vi "CRYGraph Property Window Polar.vi"(9 "TabName":string, 10 "Graph VI Ref":refnum<vi>) -> ()   [LabVIEW 2013]
uses:
  Control/CRYPolar Property.ctl
  <vilib>/Utility/miscctls.llb/LVRowAndColumnTypeDef.ctl
  CRYCurveLibrary/Global/CRYCurve Library Global.vi
panel:
  in  "Dis/RanFreqUpdate":bool
  in  "XYCursorChange":string caption="Title Name"
  in  "EndbyOK":bool
  in  "FreqUpdate":bool
  out "Scale Style":u8=5
  out "Interpolation":string
  in  "Plot PropertyCtrl Ref":refnum<vi>
  in  "Plot Property":string
  out "PointStyle":string
  out "LineWidth":string
  out "LineStyle":string
  out "CurValuesRef":refnum<vi>[](array[refnum])
  out "CruColorsRef":refnum<vi>[](array[refnum])
  in  "SetFormat":bool
  in  "No Data":bool
  in  "CurColValPlot":bool
  out "CurColors":u32[](array[numeric])
  out "CurValues":dbl[](array[numeric])
  in  "Draw":bool
  in  "Polar Property":T1={"polar attributes"={"maximum"=2.0, "minimum"=0.0, "clip to min"=FALSE, "log"=FALSE, "grid color"=3381657, "plot color"=16711680, "fmt and prec"={"format"=enum."Decimal", "precision"=2}, "visible section"=4}, "Auto/Manual"=0, "Zero Adjust (deg)"=0, "Angle Increment (deg)"=0, "Mirror"=FALSE, "Auto Increment"=FALSE, "Total Rotatin (deg)"=0, "Discrete/Rannge"=0, "Show Name"=FALSE, "CurValues"=[], "CurIndex"=0, "CurColors"=[], "CurColors_Range"=[], "CurValues_Range"=[], "Pen"={"Width"=1, "Style"=enum."Solid"}, "BackgroundColor"=0} {"polar attributes"."minimum" format="%0.2f"; "polar attributes"."maximum" format="%0.2f"}
  in  "Polar Tab":enum32{"Title", "Plot", "XY Graph"}(tab)
  in  "Background Color":u32(colorbox) caption="背景颜色"
  in  "Title Name":string caption="标题名字"
  out "CurValue0_1":bool
  in  "CurValue4":dbl format="%#.5p"
  in  "CurColor4":u32(colorbox)
  in  "CurValue3":dbl format="%#.5p"
  in  "CurColor3":u32(colorbox)
  in  "CurValue2":dbl format="%#.5p"
  in  "CurColor2":u32(colorbox)
  in  "CurValue1":dbl caption="末尾频率" format="%#.5p"
  in  "CurColor1":u32(colorbox)
  in  "Delete":bool
  in  "Add":bool
  in  "Show Name":bool caption="显示名字"
  out "Cursors":bool caption="游标"
  in  "Discrete/Range":u16(slide)
  in  "CurIndex":u16
  in  "CurValue0":dbl caption="开始频率" format="%#.5p"
  in  "CurColor0":u32(colorbox)
  out "Plot Options":bool caption="绘图选项"
  out "Scaling":bool caption="缩放"
  in  "Auto Increment":bool caption="自动增量"
  in  "Log":bool caption="对数"
  in  "Mirror":bool caption="镜子反射"
  in  "Auto/Manual":u16(slide)
  in  "Minimum":dbl caption="最小值"
  in  "Clip to min":bool caption="剪辑最低"
  in  "Angle Increment (deg)":i32 caption="角度增量(度)"
  in  "Zero Adjust (deg)":i32 caption="调零(度)"
  in  "Maximum":dbl caption="最大值"
  in  "PrecisionPolar":u8 caption="精度"
  in  "Grid Color":u32(colorbox) caption="网格颜色"
  in  "Line Width":u16(ring) caption="绘图线宽度" items=["1", "2", "3", "4", "5", "6"]
  in  "Visible Section":u16(ring)=4 caption="可见部分"
  in  "Total Rotatin (deg)":i32 caption="aa"
  in  "Line Style":u16(ring) caption="线条样式" items=["实线", "虚线", "点线", "点划线", "双点划线"]
  in  "PolarXY Tab":enum32{"Format and Precision", "Plot", "Scale"}(tab) caption="Property Tab"
  in  "FormatAxis":u16(ring) items=["Hz", "dB re 1 ", "dB re 1"]
  in  "NotationXY":i32(listbox)
  in  "PrecisionType":u16(ring) items=["精度位数", "有效数字"]
  in  "PrecisionDigits":u16
  in  "Hide trailing zeros":bool caption="隐藏尾随零"
  in  "Exponent in multiples of 3":bool caption="指数"
  in  "Use minimum field width":bool caption="使用最小场宽度"
  in  "Field Width":u16
  in  "PadType":u16(ring) items=["在左加空格", "在右加空格", "在左加零"]
  in  "Ignore timestamp information":bool caption="忽略时间戳信息"
  in  "TimeFormat":u16(ring) items=["Custom time format", "System time format", "Time unused"]
  in  "Digits":u16 caption="数字"
  in  "DateFormat":u16(ring) items=["Custom date format", "System date format", "Date unused"]
  in  "YMD":u16(slide)
  in  "YearShow":u16(slide)
  in  "AMFM":u16(slide)=1
  in  "HMS":u16(slide)=1
  in  "Point/Fill":u32(colorbox) caption="点/填充"
  in  "Fill to":i16(ring) caption="填写" items=["无"=-1, "零"=-2, "-无穷"=-3, "+无穷"=-4]
  in  "Items":u16(ring) items=["Crown Amp-R corr-out", "Crown Amp-R eq-out"]
  out "Colors":bool caption="颜色"
  in  "Line":u32(colorbox) caption="线"
  in  "LineStyle4":bool
  in  "LineStyle3":bool
  in  "LineStyle2":bool
  in  "LineStyle0":bool
  in  "LineStyle1":bool
  in  "LineWidth5":bool
  in  "LineWidth1":bool
  in  "LineWidth4":bool
  in  "LineWidth3":bool
  in  "LineWidth2":bool
  in  "LineWidth0":bool
  in  "PointStyle16":bool
  in  "PointStyle15":bool
  in  "PointStyle14":bool
  in  "PointStyle13":bool
  in  "PointStyle12":bool
  in  "PointStyle11":bool
  in  "PointStyle10":bool
  in  "PointStyle9":bool
  in  "PointStyle8":bool
  in  "PointStyle7":bool
  in  "PointStyle6":bool
  in  "PointStyle5":bool
  in  "PointStyle4":bool
  in  "PointStyle3":bool
  in  "PointStyle2":bool
  in  "PointStyle1":bool
  in  "PointStyle0":bool
  in  "Interpolation4":bool
  in  "Interpolation5":bool
  in  "Interpolation3":bool
  in  "Interpolation2":bool
  in  "Interpolation1":bool
  in  "Interpolation0":bool
  in  "Show Plot":bool caption="显示绘图"
  in  "GridStyle":u16(ring)=4
  out "Grid Colors":bool caption="网格颜色"
  in  "Minor grid":u32(colorbox) caption="辅网格"
  in  "Major grid":u32(colorbox) caption="主网格"
  in  "Marker text":u32(colorbox) caption="标记文本"
  in  "Minor tick":u32(colorbox) caption="辅刻度"
  in  "LogXY":bool caption="对数"
  in  "Show scale":bool caption="显示缩放"
  in  "Show scale label":bool caption="显示缩放标签"
  in  "MaximumXY":dbl caption="最大值"
  in  "MinimumXY":dbl caption="最小值"
  in  "Autoscale":bool caption="自动缩放"
  in  "Axis Name":string caption="名字"
  in  "Axis":u16(ring) items=["Hz", "dB re 1 ", "dB re 1"]
  in  "Major tick":u32(colorbox) caption="主刻度"
  out "Scale Style and Colors":bool caption="缩放样式和颜色"
  in  "OK":bool
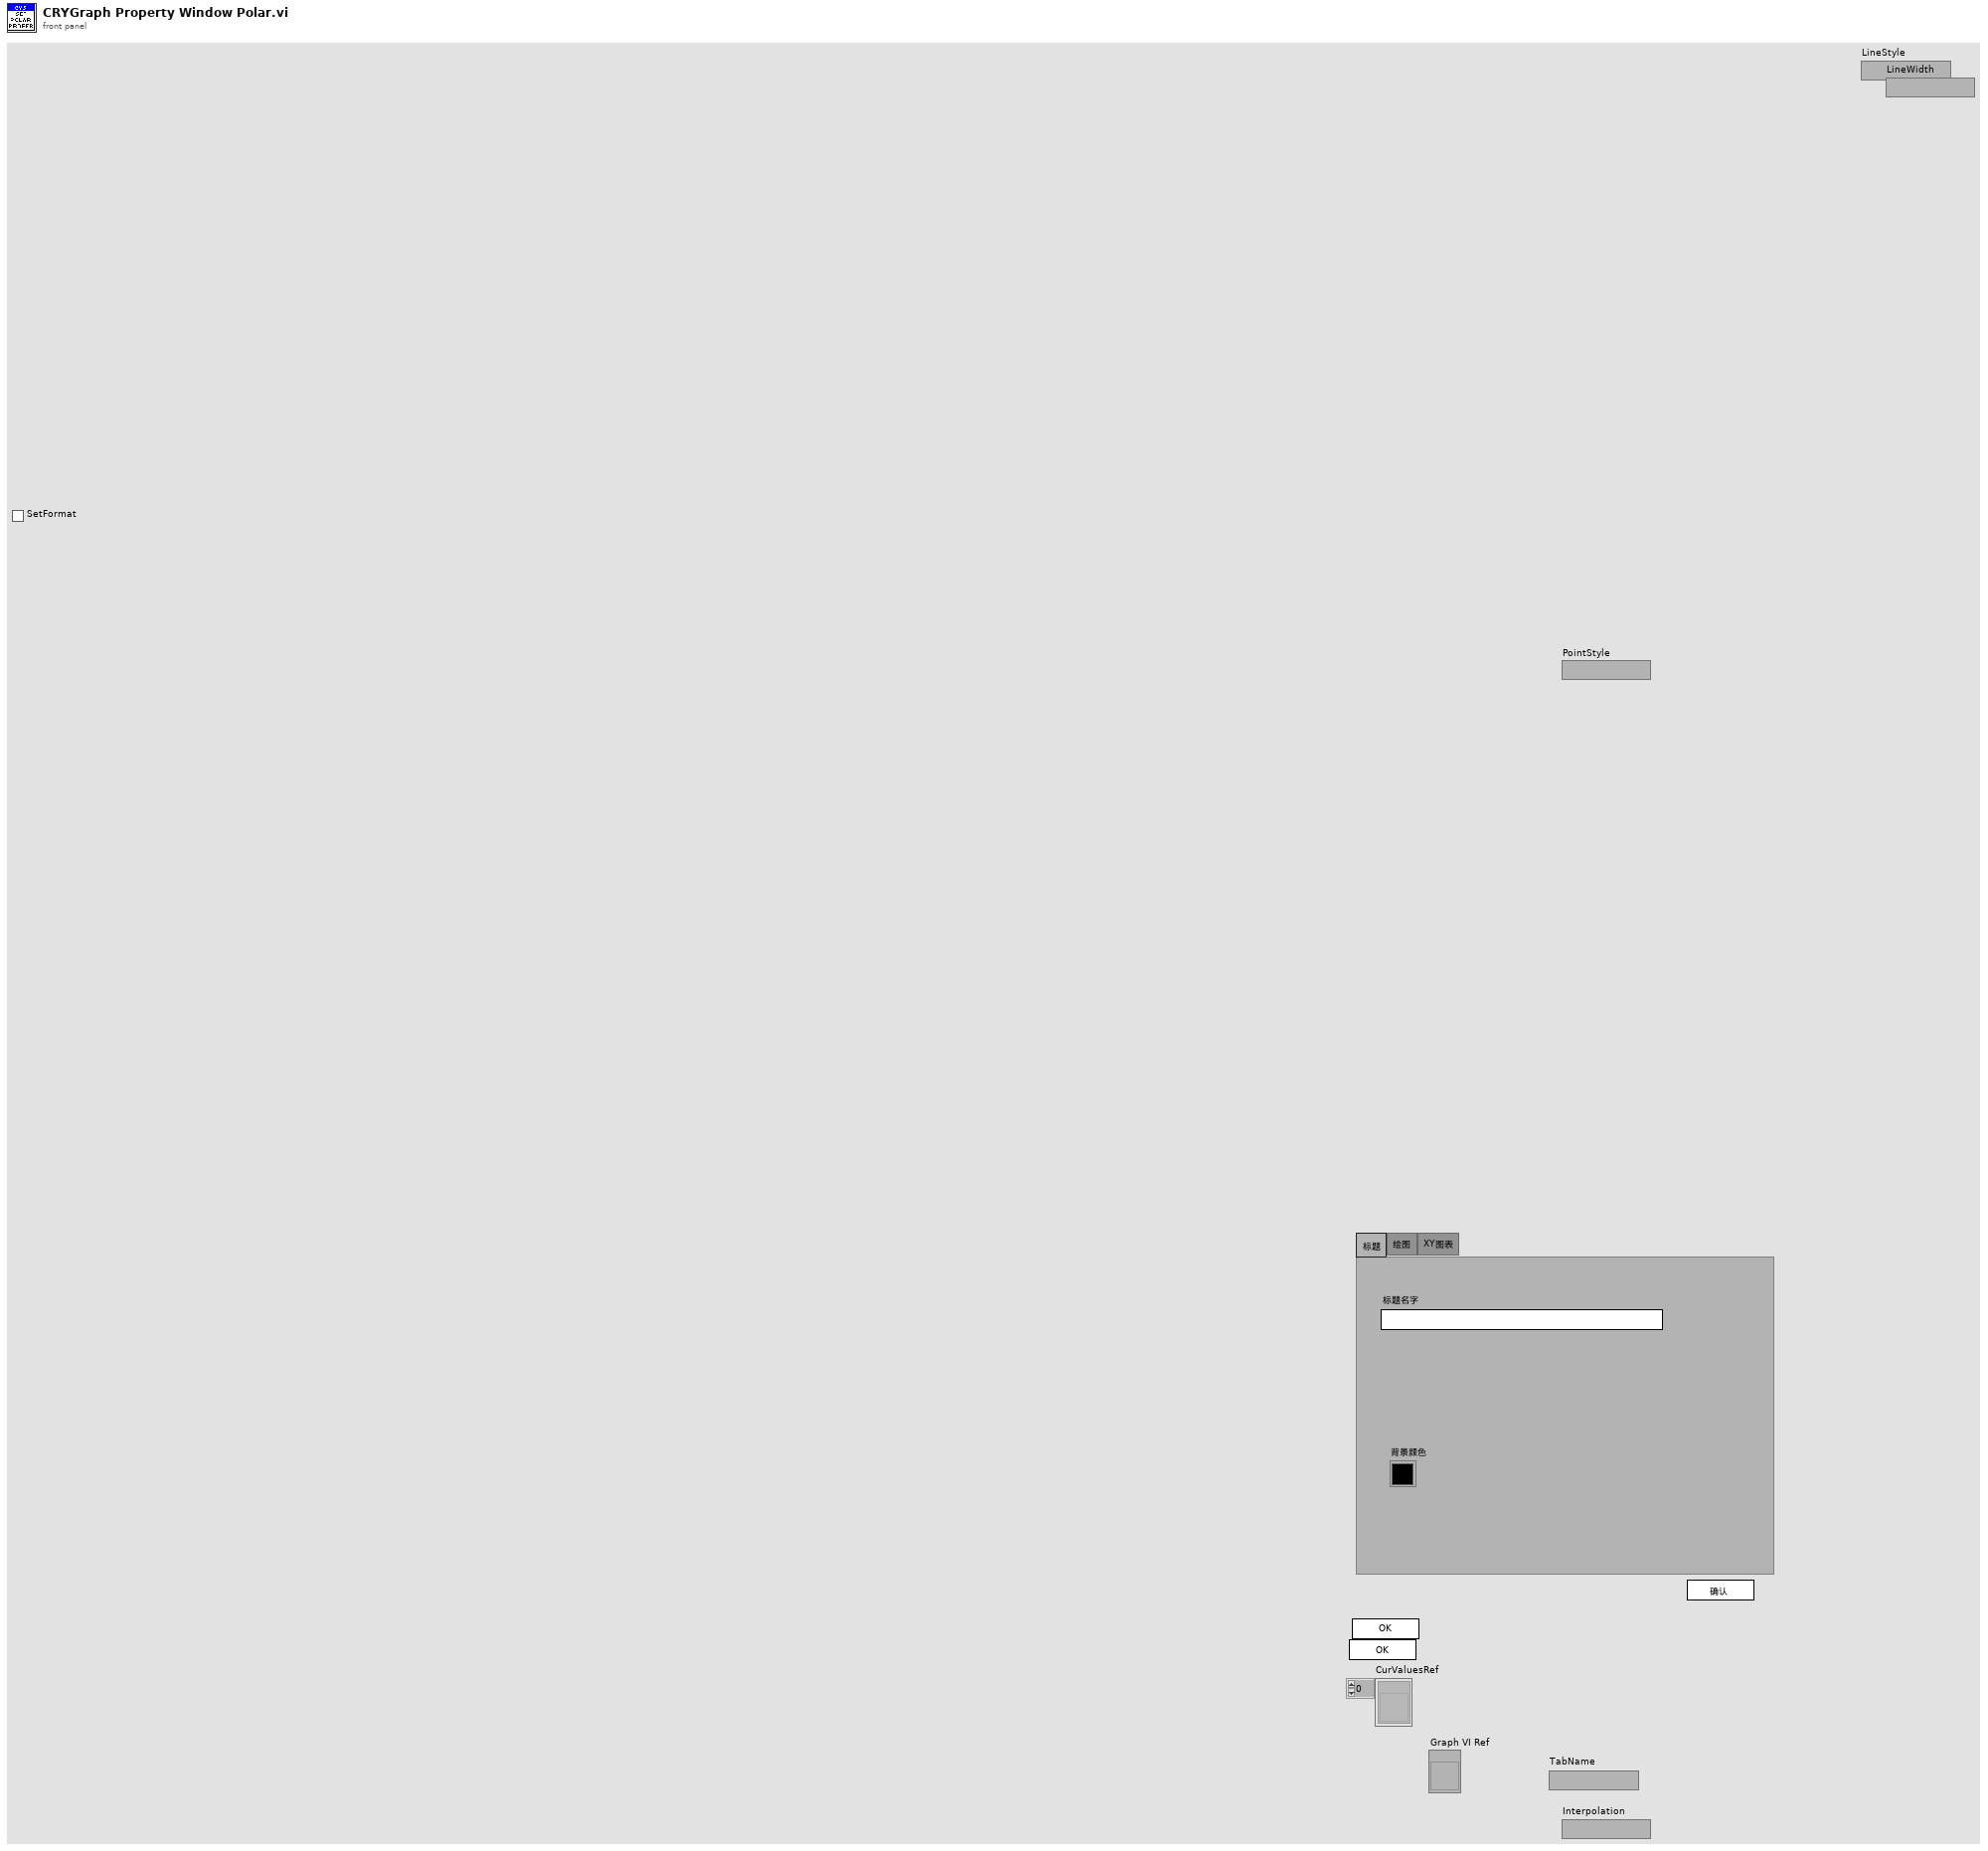
[diagram p1: front panel]
types:
  T1 = typedef "CRYPolar Property.ctl" = cluster{"polar attributes":cluster{"maximum":dbl, "minimum":dbl, "clip to min":bool, "log":bool, "grid color":u32, "plot color":u32, "fmt and prec":cluster{"format":enum8{"Decimal", "Scientific", "Engineering", "Binary", "Octal", "Hex"}, "precision":u8}, "visible section":u16}, "Auto/Manual":u16, "Zero Adjust (deg)":i32, "Angle Increment (deg)":i32, "Mirror":bool, "Auto Increment":bool, "Total Rotatin (deg)":i32, "Discrete/Rannge":u16, "Show Name":bool, "CurValues":dbl[], "CurIndex":u16, "CurColors":u32[], "CurColors_Range":u32[], "CurValues_Range":dbl[], "Pen":cluster{"Width":u16, "Style":enum32{"Solid", "Dash", "Dot", "DashDot", "DashDotDot"}}, "BackgroundColor":u32}
  T2 = enum32{"Page Enabled", "Page Disabled", "Page Disabled & Grayed"}
  T3 = enum8{"Enabled", "Disabled", "Disabled and Grayed Out"}
  T4 = typedef "LVCursorListTypeDef.ctl" = cluster{"Name":string, "Color":u32, "Style":u8, "Point Style":u8, "Name Visible":bool, "Allow Drag":bool, "Cursor Mode":u32, "Plot":i32, "Index":i32, "Position":cluster{"X":dbl, "Y":dbl}, "X Scale":u32, "Y Scale":u32, "Watch Plots":i32[], "Watch All Plots":bool, "Plot Area":i32, "Label Offset":cluster{"X":dbl, "Y":dbl}}[]
  T5 = cluster{"Width":u16, "Style":enum32{"Solid", "Dash", "Dot", "DashDot", "DashDotDot"}}
  T6 = cluster{"maximum":dbl, "minimum":dbl, "clip to min":bool, "log":bool, "grid color":u32, "plot color":u32, "fmt and prec":cluster{"format":enum8{"Decimal", "Scientific", "Engineering", "Binary", "Octal", "Hex"}, "precision":u8}, "visible section":u16}
  T7 = enum32{"Solid", "Dash", "Dot", "DashDot", "DashDotDot"}
  T8 = cluster{"format":enum8{"Decimal", "Scientific", "Engineering", "Binary", "Octal", "Hex"}, "precision":u8}
  T9 = enum16{"OK", "Yes", "YesNo", "YesNoCancel", "ReplaceAppend"}
  T10 = enum8{"Decimal", "Scientific", "Engineering", "Binary", "Octal", "Hex"}
  T11 = typedef "LVRowAndColumnTypeDef.ctl" = cluster{"Row":i32, "Column":i32}
  T12 = typedef "CRYData Cluster.ctl" = cluster{"Name":string, "Curve":cluster{"x":dbl, "y":dbl, "z":dbl}[], "X data":u16, "Y data":u16, "Z data":u16, "X axis":u16, "Y axis":u16, "Z axis":u16, "X unit":string, "Y unit":string, "Z unit":string, "X dB ref":dbl, "Y dB ref":dbl, "Z dB ref":dbl, "single val":bool, "protected":bool, "display X":bool, "display Y":bool, "display Z":bool, "Test Info":string, "Step No.":i32, "Plot Settings":cluster{"Color":u32, "Interpolation":u8, "Point Style":u8, "Line Style":u8, "Point Color":u32, "Line Width":u8, "Bar Plot Style":u8, "Fill To":i16}, "AutoProtect":bool}
  T13 = cluster{"Notation":i32, "PrecisionType":u16, "PrecisionDigits":u16, "Hide trailing zeros":bool, "Exponent in multiples of 3":bool, "Field Width":u16, "PadType":u16, "Use minimum field width":bool, "TimeFormat":u16, "AMFM":u16, "HMS":u16, "Digits":u16, "DateFormat":u16, "YMD":u16, "YearShow":u16}
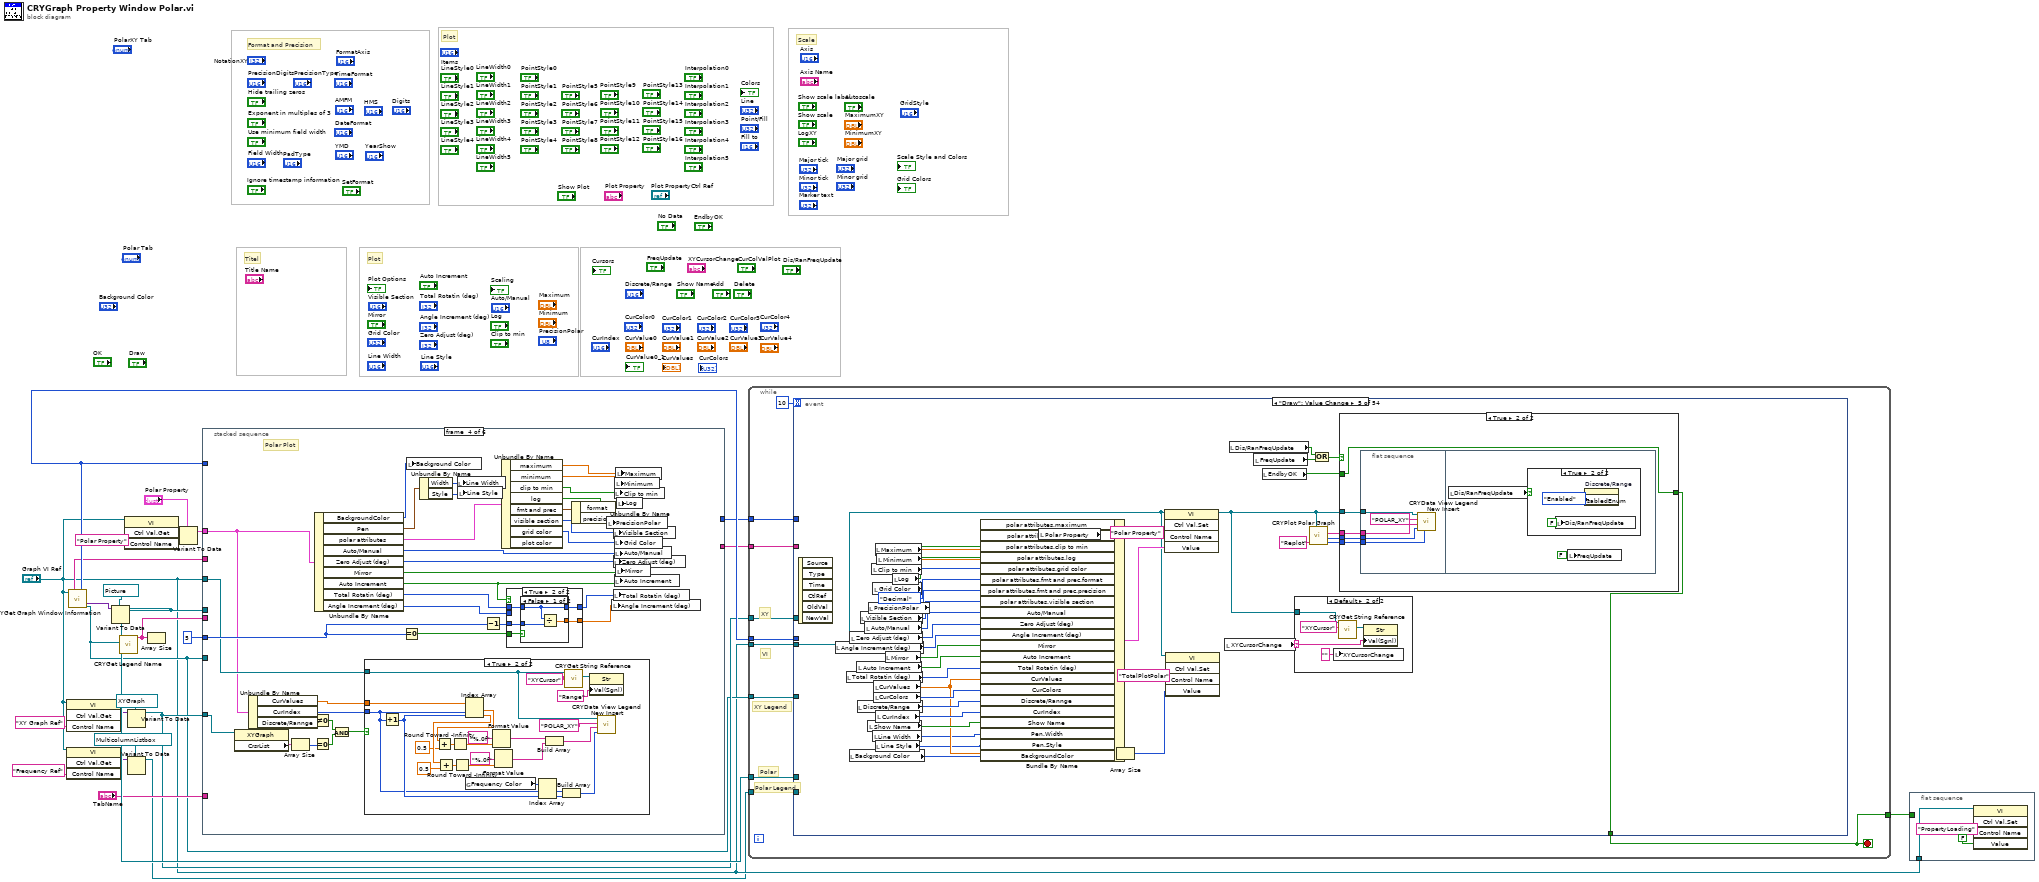
[diagram p0: block diagram]
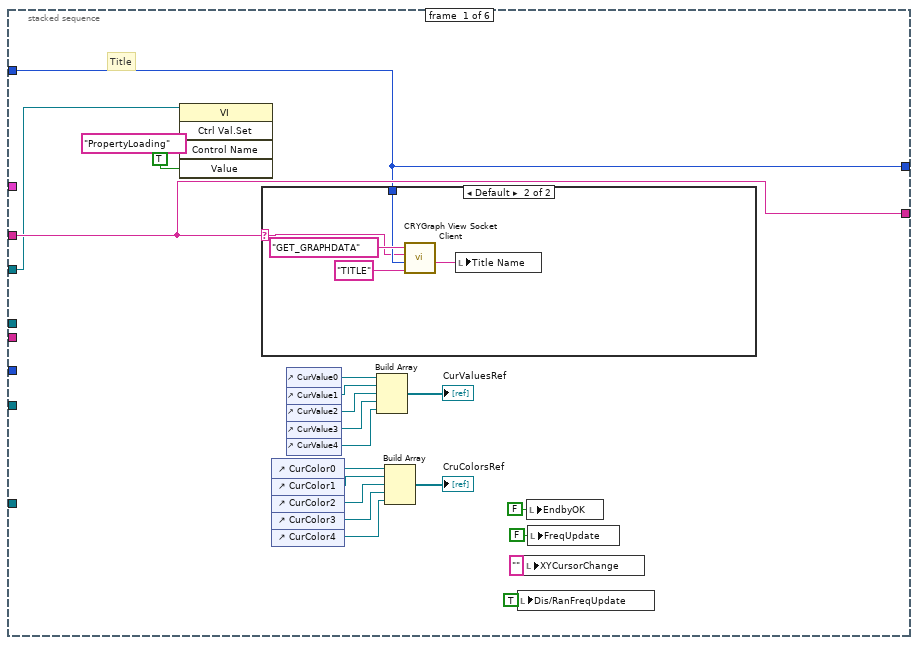
[diagram p2: hidden frame]
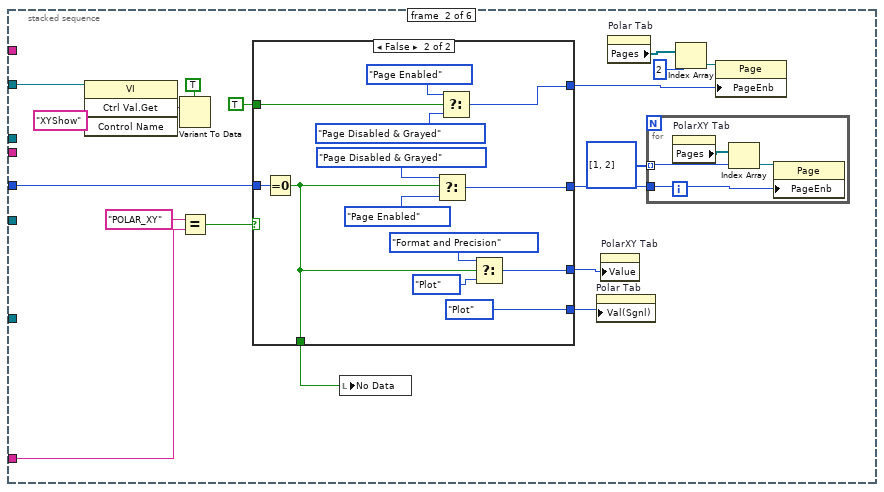
[diagram p4: hidden frame]
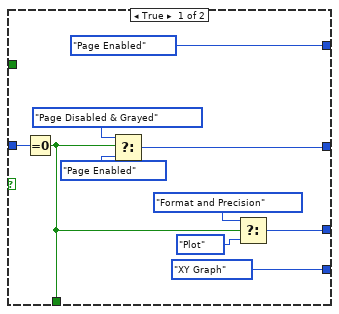
[diagram p5: hidden frame]
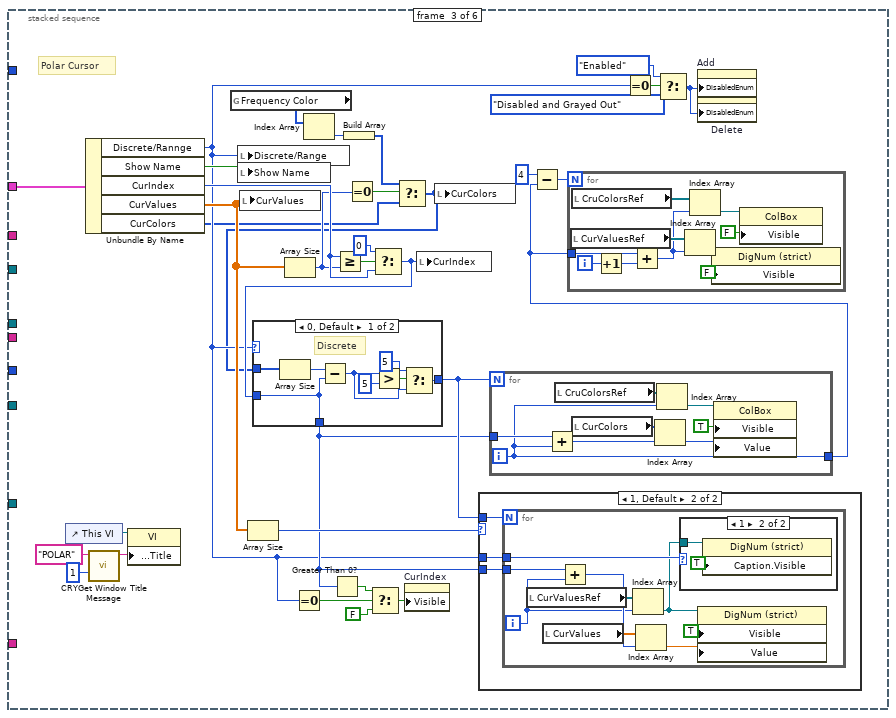
[diagram p6: hidden frame]
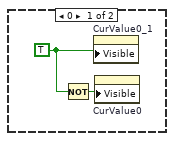
[diagram p7: hidden frame]
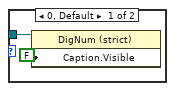
[diagram p8: hidden frame]
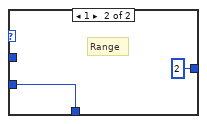
[diagram p9: hidden frame]
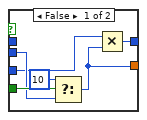
[diagram p11: hidden frame]
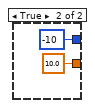
[diagram p12: hidden frame]
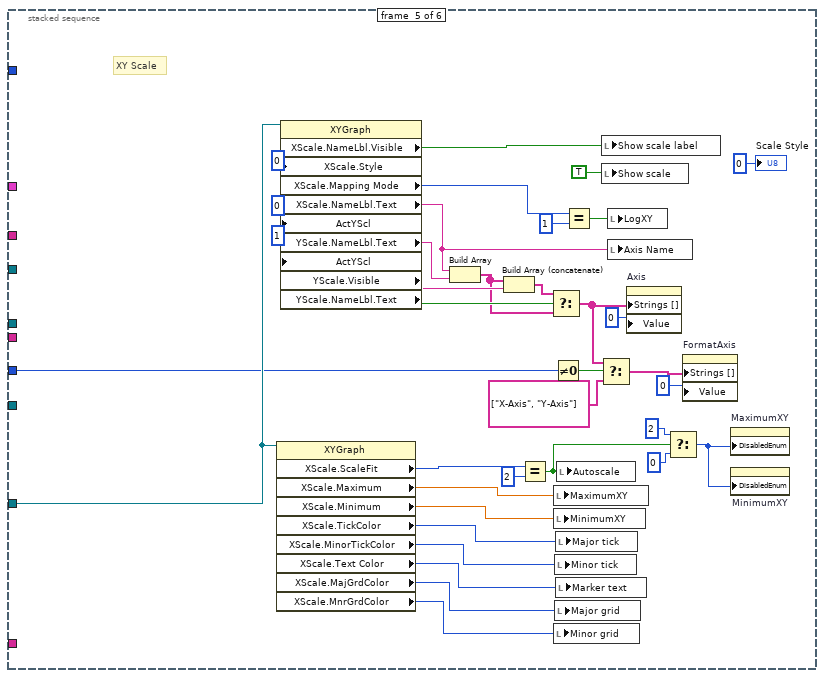
[diagram p13: hidden frame]
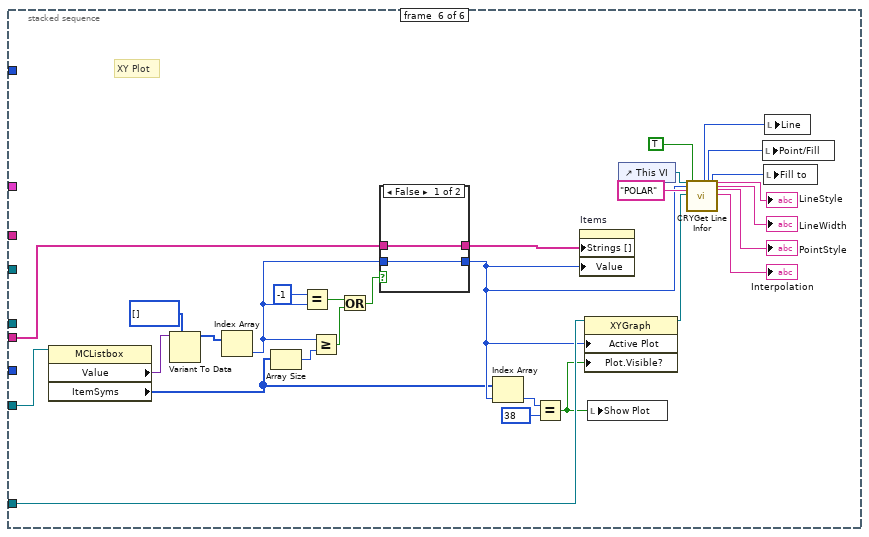
[diagram p14: hidden frame]
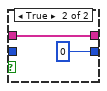
[diagram p15: hidden frame]
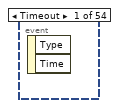
[diagram p16: hidden frame]
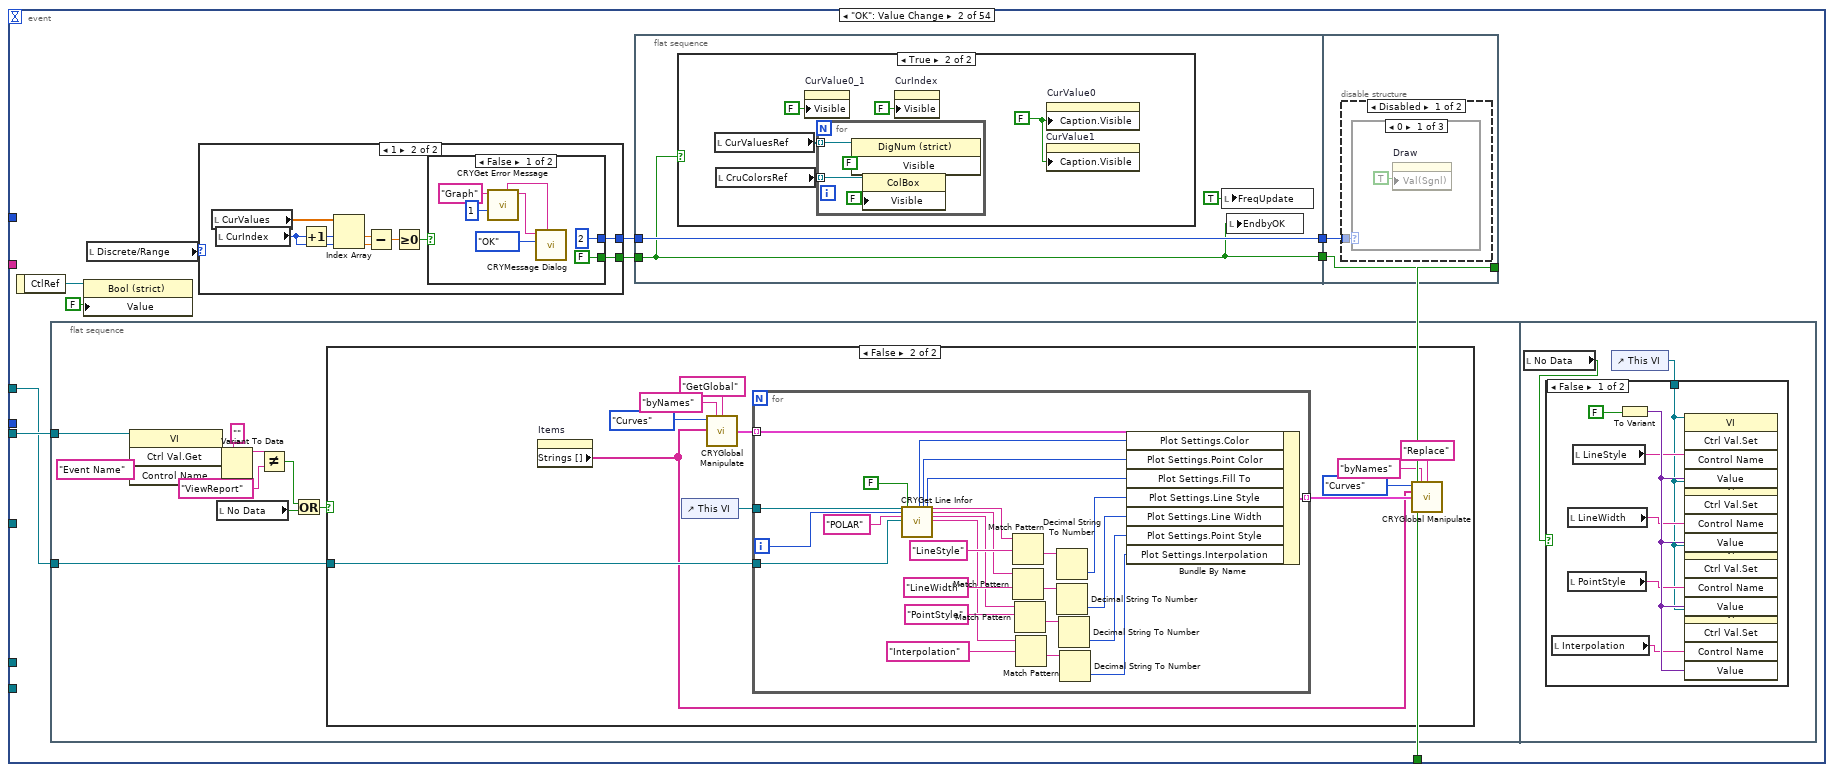
[diagram p17: hidden frame]
diagram:
  # "Format and Precision"
  # "Scale"
  # "Plot"
  # "Plot"
  # "Titel"
  n1 = invoke class="VI" method="Ctrl Val.Get"(reference="Graph VI Ref", "Control Name"="XY Graph Ref") -> ("Get Control Value Variant"=w4:variant)  [unwired: 2 in, 3 out]
  n2 = invoke class="VI" method="Ctrl Val.Get"(reference="Graph VI Ref", "Control Name"="Frequency Ref") -> ("Get Control Value Variant"=w3:variant)  [unwired: 2 in, 3 out]
  n3 = call "CRYGet Graph Window Information.vi"("pGraph VI In"="Graph VI Ref") -> ("Queue Name Out"=w23:string, "Graph Number Out"=w24:i32, "Graph Control Ref Out"=w10:variant, "Legend Ref Out"=w16:refnum<vi>)  [unwired: 2 in, 9 out]
  n4 = Variant To Data(type=refnum<vi> refnum ("Graph Ref"), Variant=w10) -> (data=w25:refnum<vi>)  [unwired: 1 in, 1 out]
  n5 = call "CRYGet Legend Name.vi"("MCListbox Refnum"=w16) -> ("Names Out"=w17:string[])  [unwired: 1 in, 9 out]
  n6 = invoke class="VI" method="Ctrl Val.Get"(reference="Graph VI Ref", "Control Name"="Polar Property") -> ("Get Control Value Variant"=w9:variant)  [unwired: 2 in, 3 out]
  n7 = Variant To Data(type=refnum<vi> refnum ("XY Graph"), Variant=w4) -> (data=w19:refnum<vi>)  [unwired: 1 in, 1 out]
  n8 = Variant To Data(type=refnum<vi> refnum ("XY Graph"), Variant=w3) -> (data=w13:refnum<vi>)  [unwired: 1 in, 1 out]
  n9 = Array Size(array=w17) -> ()  [unwired: 1 out]
  n10 = Variant To Data(type="Polar Property", Variant=w9) -> (data=w21:T1)  [unwired: 1 in, 1 out]
  n11 = stacked-sequence {
    tunnel: w25 -> [_ _ _ _ _ _]
    tunnel: w24 -> [w26 _ _ _ _ _]
    tunnel: w23 -> [w46 _ _ _ _ _]
    tunnel: [w46 _ _ _ _ _] -> w22
    tunnel: w21 -> [_ _ w129 w180 _ _]
    tunnel: "TabName" -> [_ w53 _ _ _ _]
    tunnel: "Graph VI Ref" -> [w31 w55 _ w188 _ _]
    tunnel: w19 -> [_ _ _ w187 w272 w300]
    tunnel: 5 -> [_ w54 _ w191 w253 _]
    tunnel: w17 -> [_ _ _ _ _ w302]
    tunnel: w16 -> [_ _ _ _ _ w301]
    tunnel: [w26 _ _ _ _ _] -> w12
    frame #0 {
      # "Title"
      n12 = invoke class="VI" method="Ctrl Val.Set"(reference=w31, "Control Name"="PropertyLoading", "Value"=TRUE ("FreqUpdate")) -> ()  [unwired: 2 in, 5 out]
      n13 = case shown="Default" w46 {
        selector: w46 -> [_ w48]
        tunnel: w26 -> [_ w49]
        frame "test DataView" {
        }
        frame Default {
          n14 = call "CRYGraph View Socket Client.vi"("sOption"="TITLE", "nData"=w49, "sData"=w48, "sAction"="GET_GRAPHDATA") -> ("sData Out"=w47:string)  [unwired: 4 in, 3 out]
          n15 = local write "Title Name"(w47) -> ()
        }
      }
      n16 = control-ref of="CurColor0"() -> (w45:refnum<vi>)
      n17 = control-ref of="CurColor1"() -> (w44:refnum<vi>)
      n18 = control-ref of="CurColor2"() -> (w43:refnum<vi>)
      n19 = control-ref of="CurColor3"() -> (w42:refnum<vi>)
      n20 = control-ref of="CurColor4"() -> (w41:refnum<vi>)
      n21 = control-ref of="CurValue0"() -> (w40:refnum<vi>)
      n22 = control-ref of="CurValue1"() -> (w39:refnum<vi>)
      n23 = control-ref of="CurValue2"() -> (w38:refnum<vi>)
      n24 = control-ref of="CurValue3"() -> (w37:refnum<vi>)
      n25 = control-ref of="CurValue4"() -> (w36:refnum<vi>)
      n26 = Build Array(w40, w39, w38, w37, w36) -> (→"CurValuesRef":refnum<vi>[])
      n27 = Build Array(w45, w44, w43, w42, w41) -> (→"CruColorsRef":refnum<vi>[])
      n28 = local write "Dis/RanFreqUpdate"(TRUE ("Dis/RanFreqUpdate")) -> ()
      n29 = local write "XYCursorChange"("" ("XYCursorChange")) -> ()
      n30 = local write "EndbyOK"(FALSE ("EndbyOK")) -> ()
      n31 = local write "FreqUpdate"(FALSE ("FreqUpdate")) -> ()
    }
    frame #1 {
      n32 = invoke class="VI" method="Ctrl Val.Get"(reference=w55, "Control Name"="XYShow") -> ("Get Control Value Variant"=w60:variant)  [unwired: 2 in, 3 out]
      n33 = Variant To Data(type=TRUE, Variant=w60) -> ()  [unwired: 1 in, 2 out]
      n34 = Equal?(x="POLAR_XY" ("y"), y=w53) -> (x = y?=w67:bool)
      n35 = case shown="False" w67 {
        tunnel: TRUE -> [_ w89]
        tunnel: [enum32{"Title", "Plot", "XY Graph"}."XY Graph" ("Value (Signaling)") enum32{"Title", "Plot", "XY Graph"}."Plot" ("Value (Signaling)")] -> w66
        tunnel: w54 -> [w82 w95]
        tunnel: [w79 w92] -> w65
        tunnel: [T2."Page Enabled" ("Page Enabled State") w88] -> w63
        tunnel: [w75 w85] -> w62
        tunnel: [w74 w84] -> w56
        frame True {
          n36 = Equal To 0?(x=w82) -> (x = 0?=w74:bool)
          n37 = Select(t=T2."Page Disabled & Grayed" ("Page Enabled State"), s=w74, f=T2."Page Enabled" ("Page Enabled State")) -> (s? t:f=w79:T2)
          n38 = Select(t=enum32{"Format and Precision", "Plot", "Scale"}."Format and Precision" ("XY Tab"), s=w74, f=enum32{"Format and Precision", "Plot", "Scale"}."Plot" ("XY Tab")) -> (s? t:f=w75:enum32{"Format and Precision", "Plot", "Scale"})
        }
        frame False {
          n39 = Equal To 0?(x=w95) -> (x = 0?=w84:bool)
          n40 = Select(t=T2."Page Disabled & Grayed" ("Page Enabled State"), s=w84, f=T2."Page Enabled" ("Page Enabled State")) -> (s? t:f=w92:T2)
          n41 = Select(t=T2."Page Enabled" ("Page Enabled State"), s=w89, f=T2."Page Disabled & Grayed" ("Page Enabled State")) -> (s? t:f=w88:T2)
          n42 = Select(t=enum32{"Format and Precision", "Plot", "Scale"}."Format and Precision" ("XY Tab"), s=w84, f=enum32{"Format and Precision", "Plot", "Scale"}."Plot" ("XY Tab")) -> (s? t:f=w85:enum32{"Format and Precision", "Plot", "Scale"})
        }
      }
      n43 = local write "No Data"(w56) -> ()
      n44 = property on="Polar Tab" class="TabCtl (strict)"("Val(Sgnl)"=w66) -> ()  [unwired: 2 in, 2 out]
      n45 = property on="PolarXY Tab" class="TabCtl (strict)"("Value"=w62) -> ()  [unwired: 2 in, 2 out]
      n46 = property on="Polar Tab" class="TabCtl (strict)"() -> ("Pages"=w69:refnum<vi>[])  [unwired: 2 in, 2 out]
      n47 = for {
        tunnel: w65 -> [w71]
        tunnel: i32[] [1, 2] -> [w70] mode=indexing
        n48 = property on="PolarXY Tab" class="TabCtl (strict)"() -> ("Pages"=w72:refnum<vi>[])  [unwired: 2 in, 2 out]
        n49 = Index Array(array=w72, index=w70) -> (element=w73:refnum<vi>)
        n50 = property class="Page"(reference=w73, "PageEnb"=w71) -> ()  [unwired: 1 in, 2 out]
      }
      n51 = Index Array(array=w69, index=2) -> (element=w68:refnum<vi>)
      n52 = property class="Page"(reference=w68, "PageEnb"=w63) -> ()  [unwired: 1 in, 2 out]
    }
    frame #2 {
      # "Polar Cursor"
      n53 = control-ref of="This VI"() -> (w128:refnum<vi>)
      n54 = Unbundle By Name(w129) -> ("Discrete/Rannge"=w108:u16, "Show Name"=w114:bool, "CurIndex"=w110:u16, "CurValues"=w113:dbl[], "CurColors"=w98:u32[])
      n55 = call "CRYGet Window Title Message.vi"("No"=1 ("Error No"), "Kind"="POLAR") -> ("Multibyte String"=w127:string)  [unwired: 4 in, 5 out]
      n56 = property class="VI"(reference=w128, "Front Panel.Title"=w127) -> ()  [unwired: 1 in, 2 out]
      n57 = global read "CRYCurve Library Global.vi" "Frequency Color"() -> (w103:u32[])
      n58 = local write "Discrete/Range"(w108) -> ()
      n59 = local write "Show Name"(w114) -> ()
      n60 = local write "CurValues"(w113) -> ()
      n61 = Array Size(array=w113) -> (size(s)=w121:i32)
      n62 = Array Size(array=w113) -> (size(s)=w101:i32)
      n63 = Equal To 0?(x=w108) -> (x = 0?=w107:bool)
      n64 = Index Array(array=w103) -> (element=w102:u32)  [unwired: 1 in]
      n65 = Greater Or Equal?(x=w110, y=w101) -> (x >= y?=w112:bool)
      n66 = Build Array(w102) -> (w99:u32[])
      n67 = Equal To 0?(x=w101) -> (x = 0?=w100:bool)
      n68 = Select(t=u16 0 ("CurIndex"), s=w112, f=w110) -> (s? t:f=w109:u16)
      n69 = Select(t=w99, s=w100, f=w98) -> (s? t:f=w97:u32[])
      n70 = case shown="0, Default" w108 {
        tunnel: [w163 2 ("y")] -> w120
        tunnel: [w159 w166] -> w119
        tunnel: w109 -> [w159 w166]
        tunnel: w97 -> [w158 _]
        frame 0, Default {
          # "Discrete"
          n71 = Array Size(array=w158) -> (size(s)=w161:i32)
          n72 = Subtract(x=w161, y=w159) -> (x-y=w162:i32)
          n73 = Greater?(x=w162, y=5) -> (0:w160:bool)
          n74 = Select(t=5 ("y"), s=w160, f=w162) -> (s? t:f=w163:i32)
        }
        frame 1 {
          # "Range"
        }
      }
      n75 = Greater Than 0?(x=w119) -> (x > 0?=w104:bool)
      n76 = Select(t=w104, s=w107, f=FALSE ("Visible")) -> (s? t:f=w105:bool)
      n77 = property on="CurIndex" class="DigNum (strict)"("Visible"=w105) -> ()  [unwired: 2 in, 2 out]
      n78 = local write "CurIndex"(w109) -> ()
      n79 = local write "CurColors"(w97) -> ()
      n80 = case shown="1, Default" w121 {
        tunnel: w108 -> [_ w134]
        tunnel: w119 -> [_ w133]
        tunnel: w120 -> [_ w132]
        frame 0 {
          w130 = TRUE ("Value (Signaling)")
          n81 = Not(x=w130) -> (.not. x?=w131:bool)
          n82 = property on="CurValue0_1" class="Bool (strict)"("Visible"=w130) -> ()  [unwired: 2 in, 2 out]
          n83 = property on="CurValue0" class="DigNum (strict)"("Visible"=w131) -> ()  [unwired: 2 in, 2 out]
        }
        frame 1, Default {
          n84 = for {
            N: w132 -> [_]
            tunnel: w133 -> [w142]
            tunnel: w134 -> [w136]
            i -> [w137]
            n85 = local read "CurValuesRef"() -> (w139:refnum<vi>[])
            n86 = local read "CurValues"() -> (w143:dbl[])
            n87 = Add(x=w142, y=w137) -> (x+y=w138:i32)
            n88 = Index Array(array=w139, index=w137) -> (element=w135:refnum<vi>)
            n89 = Index Array(array=w143, index=w138) -> (element=w141:dbl)
            n90 = case shown="1" w136 {
              tunnel: w135 -> [w144 w146]
              frame 0, Default {
                n91 = property class="DigNum (strict)"(reference=w144, "Caption.Visible"=FALSE ("Label.Visible")) -> ()  [unwired: 1 in, 2 out]
              }
              frame 1 {
                n92 = property class="DigNum (strict)"(reference=w146, "Caption.Visible"=TRUE ("Label.Visible")) -> ()  [unwired: 1 in, 2 out]
              }
            }
            n93 = property class="DigNum (strict)"(reference=w135, "Visible"=TRUE, "Value"=w141) -> ()  [unwired: 1 in, 2 out]
          }
        }
      }
      n94 = for {
        N: w120 -> [_]
        tunnel: w119 -> [w174]
        tunnel: [w169] -> w122
        i -> [w169]
        n95 = Add(x=w174, y=w169) -> (x+y=w170:i32)
        n96 = local read "CruColorsRef"() -> (w171:refnum<vi>[])
        n97 = local read "CurColors"() -> (w175:u32[])
        n98 = Index Array(array=w175, index=w170) -> (element=w173:u32)
        n99 = Index Array(array=w171, index=w169) -> (element=w168:refnum<vi>)
        n100 = property class="ColBox"(reference=w168, "Visible"=TRUE, "Value"=w173) -> ()  [unwired: 1 in, 2 out]
      }
      n101 = Subtract(x=4, y=w122) -> (x-y=w124:i32)
      n102 = for {
        N: w124 -> [_]
        tunnel: w122 -> [w154]
        i -> [w156]
        n103 = local read "CurValuesRef"() -> (w151:refnum<vi>[])
        n104 = local read "CruColorsRef"() -> (w152:refnum<vi>[])
        n105 = Increment(x=w156) -> (x+1=w155:i32)
        n106 = Add(x=w154, y=w155) -> (x+y=w150:i32)
        n107 = Index Array(array=w151, index=w150) -> (element=w148:refnum<vi>)
        n108 = Index Array(array=w152, index=w150) -> (element=w149:refnum<vi>)
        n109 = property class="DigNum (strict)"(reference=w148, "Visible"=FALSE) -> ()  [unwired: 1 in, 2 out]
        n110 = property class="ColBox"(reference=w149, "Visible"=FALSE) -> ()  [unwired: 1 in, 2 out]
      }
      n111 = Equal To 0?(x=w108) -> (x = 0?=w115:bool)
      n112 = Select(t=T3."Enabled" ("Disabled"), s=w115, f=T3."Disabled and Grayed Out") -> (s? t:f=w118:T3)
      n113 = property on="Add" class="Bool (strict)"("DisabledEnum"=w118) -> ()  [unwired: 2 in, 2 out]
      n114 = property on="Delete" class="Bool (strict)"("DisabledEnum"=w118) -> ()  [unwired: 2 in, 2 out]
    }
    frame #3 {
      # "Polar Plot"
      n115 = property class="XYGraph"(reference=w187) -> ("CrsrList"=w186:T4)  [unwired: 1 in, 2 out]
      n116 = Unbundle By Name(w180) -> ("CurValues"=w189:dbl[], "CurIndex"=w190:u16, "Discrete/Rannge"=w184:u16)
      n117 = Array Size(array=w186) -> (size(s)=w185:i32)
      n118 = Not Equal To 0?(x=w184) -> (x != 0?=w183:bool)
      n119 = Equal To 0?(x=w185) -> (x = 0?=w182:bool)
      n120 = Unbundle By Name(w180) -> ("BackgroundColor"=w176:u32, "Pen"=w179:T5, "polar attributes"=w210:T6, "Auto/Manual"=w201:u16, "Zero Adjust (deg)"=w200:i32, "Mirror"=w199:bool, "Auto Increment"=w197:bool, "Total Rotatin (deg)"=w196:i32, "Angle Increment (deg)"=w195:i32)
      n121 = And(x=w183, y=w182) -> (x .and. y?=w181:bool)
      n122 = case shown="True" w181 {
        tunnel: w190 -> [_ w234]
        tunnel: w189 -> [_ w222]
        tunnel: w188 -> [_ w211]
        frame False {
        }
        frame True {
          n123 = Increment(x=w234) -> (x+1=w235:u16)
          n124 = global read "CRYCurve Library Global.vi" "Frequency Color"() -> (w217:u32[])
          n125 = Index Array(array=w222, index #1=w234, index #2=w235) -> (element #1=w221:dbl, element #2=w231:dbl)
          n126 = Add(x=w221, y=0.5) -> (x+y=w224:dbl)
          n127 = Add(x=w231, y=0.5) -> (x+y=w229:dbl)
          n128 = Round Toward -Infinity(1:w224) -> (0:w223:dbl)
          n129 = Round Toward -Infinity(1:w229) -> (0:w230:dbl)
          n130 = Format Value(format string="%.0f", value (0)=w223) -> (output string=w232:string)  [unwired: 1 in]
          n131 = Format Value(format string="%.0f", value (0)=w230) -> (output string=w233:string)  [unwired: 1 in]
          n132 = Index Array(array=w217, index #1=w234, index #2=w235) -> (element #1=w218:u32, element #2=w219:u32)
          n133 = Build Array(w232, w233) -> (w215:string[])
          n134 = Build Array(w218, w219) -> (w220:u32[])
          n135 = call "CRYGet String Reference.vi"("Label Name"="XYCursor", "VI Refnum"=w211) -> ("String Ref Out"=w213:refnum<vi>)  [unwired: 7 in, 2 out]
          n136 = property class="Str"(reference=w213, "Val(Sgnl)"="Range" ("Value (Signaling)")) -> ()  [unwired: 1 in, 2 out]
          n137 = call "CRYData View Legend New Insert.vi"("Color Array"=w220, "ItemName Array"=w215, "sOption"="POLAR_XY", "pGraph VI In"=w211) -> ()  [unwired: 1 in, 7 out]
        }
      }
      n138 = Equal To 0?(x=w191) -> (x = 0?=w192:bool)
      n139 = local write "Background Color"(w176) -> ()
      n140 = Unbundle By Name(w179) -> ("Width"=w178:u16, "Style"=w177:T7)
      n141 = local write "Line Width"(w178) -> ()
      n142 = local write "Line Style"(w177) -> ()
      n143 = Decrement(x=w191) -> (x-1=w198:i32)
      n144 = Unbundle By Name(w210) -> ("maximum"=w208:dbl, "minimum"=w207:dbl, "clip to min"=w206:bool, "log"=w205:bool, "fmt and prec"=w209:T8, "visible section"=w203:u16, "grid color"=w202:u32)  [unwired: 1 out]
      n145 = case shown="True" w197 {
        tunnel: w198 -> [w237 w246]
        tunnel: w196 -> [_ w245]
        tunnel: w195 -> [w239 _]
        tunnel: [w241 w242] -> w194
        tunnel: [w236 w244] -> w193
        tunnel: w192 -> [w240 w243]
        frame False {
          n146 = Select(t=10, s=w240, f=w239) -> (s? t:f=w236:i32)
          n147 = Multiply(x=w237, y=w236) -> (x*y=w241:i32)
        }
        frame True {
          n148 = case shown="False" w243 {
            tunnel: w246 -> [w249 _]
            tunnel: w245 -> [w247 _]
            tunnel: [w248 10.0] -> w244
            tunnel: [w247 -10 ("Total Rotatin (deg)")] -> w242
            frame False {
              n149 = Divide(x=w247, y=w249) -> (x/y=w248:dbl)
            }
            frame True {
            }
          }
        }
      }
      n150 = Unbundle By Name(w209) -> ("precision"=w204:u8)  [unwired: 1 out]
      n151 = local write "PrecisionPolar"(w204) -> ()
      n152 = local write "Angle Increment (deg)"(w193) -> ()
      n153 = local write "Visible Section"(w203) -> ()
      n154 = local write "Zero Adjust (deg)"(w200) -> ()
      n155 = local write "Total Rotatin (deg)"(w194) -> ()
      n156 = local write "Clip to min"(w206) -> ()
      n157 = local write "Grid Color"(w202) -> ()
      n158 = local write "Auto/Manual"(w201) -> ()
      n159 = local write "Auto Increment"(w197) -> ()
      n160 = local write "Minimum"(w207) -> ()
      n161 = local write "Maximum"(w208) -> ()
      n162 = local write "Mirror"(w199) -> ()
      n163 = local write "Log"(w205) -> ()
    }
    frame #4 {
      # "XY Scale"
      n164 = property class="XYGraph"(reference=w272) -> ("XScale.ScaleFit"=w281:u8, "XScale.Maximum"=w269:dbl, "XScale.Minimum"=w268:dbl, "XScale.TickColor"=w267:u32, "XScale.MinorTickColor"=w266:u32, "XScale.Text Color"=w265:u32, "XScale.MajGrdColor"=w264:u32, "XScale.MnrGrdColor"=w263:u32)  [unwired: 1 in, 2 out]
      n165 = property class="XYGraph"(reference=w272, "XScale.Style"=u8 0 ("X Scale.Style"), "ActYScl"=0 ("Active Y Scale"), "ActYScl"=1 ("Active Y Scale")) -> ("XScale.NameLbl.Visible"=w260:bool, "XScale.Mapping Mode"=w287:u8, "XScale.NameLbl.Text"=w259:string, "YScale.NameLbl.Text"=w284:string, "YScale.Visible"=w277:bool, "YScale.NameLbl.Text"=w276:string)  [unwired: 1 in, 2 out]
      n166 = Build Array(w259, w284) -> (w274:string[])
      n167 = Build Array (concatenate)(w274, w276) -> (w275:string[])
      n168 = Equal?(x=w281, y=u8 2 ("X Scale.Scale Fit")) -> (x = y?=w270:bool)
      n169 = Select(t=w275, s=w277, f=w274) -> (s? t:f=w257:string[])
      n170 = Not Equal To 0?(x=w253) -> (x != 0?=w252:bool)
      n171 = local write "MaximumXY"(w269) -> ()
      n172 = local write "MinimumXY"(w268) -> ()
      n173 = local write "Minor grid"(w263) -> ()
      n174 = local write "Minor tick"(w266) -> ()
      n175 = local write "Major grid"(w264) -> ()
      n176 = local write "Major tick"(w267) -> ()
      n177 = local write "Marker text"(w265) -> ()
      n178 = local write "Autoscale"(w270) -> ()
      n179 = Equal?(x=w287, y=u8 1) -> (x = y?=w262:bool)
      n180 = Select(t=w257, s=w252, f=string[] ["X-Axis", "Y-Axis"]) -> (s? t:f=w255:string[])
      n181 = local write "Show scale label"(w260) -> ()
      n182 = local write "Show scale"(TRUE ("Show scale")) -> ()
      n183 = local write "LogXY"(w262) -> ()
      n184 = local write "Axis Name"(w259) -> ()
      n185 = property on="Axis" class="Ring (strict)"("Strings []"=w257, "Value"=u16 0) -> ()  [unwired: 2 in, 2 out]
      n186 = Select(t=u8 2 ("X Scale.Scale Fit"), s=w270, f=u8 0 ("X Scale.Scale Fit")) -> (s? t:f=w258:u8)
      n187 = property on="FormatAxis" class="Ring (strict)"("Strings []"=w255, "Value"=u16 0) -> ()  [unwired: 2 in, 2 out]
      n188 = property on="MaximumXY" class="DigNum (strict)"("DisabledEnum"=w258) -> ()  [unwired: 2 in, 2 out]
      n189 = property on="MinimumXY" class="DigNum (strict)"("DisabledEnum"=w258) -> ()  [unwired: 2 in, 2 out]
      "Scale Style" <- u8 0 ("Scale Style")
    }
    frame #5 {
      # "XY Plot"
      n190 = property class="MCListbox"(reference=w301) -> ("Value"=w306:variant, "ItemSyms"=w288:i32[])  [unwired: 1 in, 2 out]
      n191 = Variant To Data(type=i32[] [], Variant=w306) -> (data=w295:i32[])  [unwired: 1 in, 1 out]
      n192 = Index Array(array=w295) -> (element=w289:i32)  [unwired: 1 in]
      n193 = Array Size(array=w288) -> (size(s)=w293:i32)
      n194 = Equal?(x=-1, y=w289) -> (x = y?=w292:bool)
      n195 = Greater Or Equal?(x=w289, y=w293) -> (x >= y?=w291:bool)
      n196 = Or(x=w292, y=w291) -> (x .or. y?=w290:bool)
      n197 = case shown="False" w290 {
        tunnel: w302 -> [w318 w320]
        tunnel: [w318 w320] -> w303
        tunnel: [w317 0 ("Data View Index")] -> w297
        tunnel: w289 -> [w317 _]
        frame False {
        }
        frame True {
        }
      }
      n198 = Index Array(array=w288, index=w297) -> (element=w305:i32)
      n199 = Equal?(x=w305, y=38) -> (x = y?=w299:bool)
      n200 = property on="Items" class="Ring (strict)"("Strings []"=w303, "Value"=w297) -> ()  [unwired: 2 in, 2 out]
      n201 = property class="XYGraph"(reference=w300, "Active Plot"=w297, "Plot.Visible?"=w299) -> (reference out=w298:refnum<vi>)  [unwired: 1 in, 1 out]
      n202 = local write "Show Plot"(w299) -> ()
      n203 = control-ref of="This VI"() -> (w314:refnum<vi>)
      n204 = call "CRYGet Line Infor.vi"("This VI"=w314, "Active Plot Number"=w297, "Graph Type"="POLAR", "XY Graph Control Ref"=w298, "Property Set?"=TRUE) -> ("Line"=w313:u32, "Point/Fill"=w312:u32, "Fill to"=w311:i16, "LineStyle"=→"LineStyle":string, "LineWidth"=→"LineWidth":string, "PointStyle"=→"PointStyle":string, "Interpolation"=→"Interpolation":string)  [unwired: 16 in]
      n205 = local write "Point/Fill"(w312) -> ()
      n206 = local write "Fill to"(w311) -> ()
      n207 = local write "Line"(w313) -> ()
    }
  }
  n208 = while {
    tunnel: w25 -> [w330]
    tunnel: w24 -> [w329]
    tunnel: "Graph VI Ref" -> [w328]
    tunnel: w16 -> [w326]
    tunnel: w22 -> [w325]
    tunnel: w19 -> [w324]
    tunnel: w13 -> [w323]
    tunnel: [w322] -> w15
    tunnel: w12 -> [w321]
    stop <- w322 stop-if-true
    # "Polar Legend"
    # "XY"
    # "XY Legend"
    # "Polar"
    # "VI"
    n209 = event shown="[4] \"Draw\": Value Change" {
      selector: _ -> [_ _ _ _ _ _ _ _ _ _ _ _ _ _ _ _ _ _ _ _ _ _ _ _ _ _ _ _ _ _ _ _ _ _ _ _ _ _ _ _ _ _ _ _ _ _ _ _ _ _ _ _ _ _]
      dyn-events: _ -> [_ _ _ _ _ _ _ _ _ _ _ _ _ _ _ _ _ _ _ _ _ _ _ _ _ _ _ _ _ _ _ _ _ _ _ _ _ _ _ _ _ _ _ _ _ _ _ _ _ _ _ _ _ _]
      timeout: 10 -> [_ _ _ _ _ _ _ _ _ _ _ _ _ _ _ _ _ _ _ _ _ _ _ _ _ _ _ _ _ _ _ _ _ _ _ _ _ _ _ _ _ _ _ _ _ _ _ _ _ _ _ _ _ _]
      tunnel: w330 -> [_ _ _ _ _ _ _ _ _ _ _ _ _ _ _ _ _ _ _ _ _ _ _ _ _ _ _ _ _ _ _ _ _ _ _ _ _ _ _ _ _ _ _ _ _ _ _ _ _ _ _ _ _ _]
      tunnel: w329 -> [_ _ _ _ _ _ _ _ _ _ _ _ _ _ _ _ _ _ _ _ _ _ _ _ _ _ _ _ _ _ _ _ _ _ _ _ _ _ _ _ _ _ _ _ _ _ _ _ _ _ _ _ _ _]
      tunnel: w328 -> [_ w333 _ _ w462 _ _ _ _ _ _ w548 w603 w638 _ _ _ w758 _ _ _ _ _ _ _ _ _ _ _ _ _ _ _ _ _ _ _ _ _ _ _ _ _ _ _ _ _ _ _ _ _ _ _ _]
      tunnel: w326 -> [_ _ _ _ _ _ _ w512 w521 _ _ _ _ _ _ _ _ _ _ _ _ _ _ _ _ _ _ _ _ _ _ _ _ _ _ w1080 w1111 w1123 w1133 w1143 _ _ _ _ _ _ _ _ _ _ _ _ _ _]
      tunnel: w325 -> [_ _ _ w445 _ _ _ _ _ _ _ _ _ _ _ _ _ _ _ _ _ _ _ _ _ _ _ _ _ _ _ _ _ _ _ _ w1110 w1124 w1134 _ _ _ _ _ _ _ _ _ _ _ _ _ _ _]
      tunnel: w324 -> [_ w331 _ _ _ _ _ _ _ _ _ _ _ _ _ _ _ _ _ w825 _ _ _ _ _ _ _ _ _ w909 _ _ _ _ _ w1082 w1113 w1126 w1135 w1144 w1169 w1219 w1231 w1241 w1259 w1274 w1284 w1295 w1306 w1317 w1328 w1339 w1374 w1385]
      tunnel: w323 -> [_ _ _ _ _ _ _ _ _ _ _ w549 _ _ _ _ _ _ _ _ _ _ _ _ _ _ _ _ _ _ _ _ _ _ _ _ _ _ _ _ _ _ _ _ _ _ _ _ _ _ _ _ _ _]
      tunnel: [_ w332 _ _ w455 _ _ _ _ _ _ _ _ _ _ _ _ _ _ _ _ _ _ _ _ _ _ _ _ _ _ _ _ _ _ _ _ _ _ _ _ _ _ _ _ _ _ _ _ _ _ _ _ _] -> w322
      tunnel: w321 -> [_ _ _ w446 _ _ _ _ _ _ _ _ _ _ _ _ _ _ _ _ _ _ _ _ _ _ _ _ _ _ _ _ _ _ _ _ _ _ _ _ _ _ _ _ _ _ _ _ _ _ _ _ _ _]
      event Timeout {
        n210 = event-data() -> ()  [unwired: 3 out]
      }
      event "OK": Value Change {
        n211 = event-data() -> ("CtlRef"=w338:refnum<vi>)  [unwired: 1 out]
        n212 = flat-sequence {
          tunnel: w333 -> [w343]
          tunnel: w331 -> [w341]
          frame #0 {
            n213 = invoke class="VI" method="Ctrl Val.Get"(reference=w343, "Control Name"="Event Name") -> ("Get Control Value Variant"=w346:variant)  [unwired: 2 in, 3 out]
            n214 = local read "No Data"() -> (w350:bool)
            n215 = Variant To Data(type="" ("Control Name"), Variant=w346) -> (data=w348:string)  [unwired: 1 in, 1 out]
            n216 = Not Equal?(x=w348, y="ViewReport" ("regular expression")) -> (x != y?=w344:bool)
            n217 = Or(x=w344, y=w350) -> (x .or. y?=w342:bool)
            n218 = case shown="False" w342 {
              tunnel: w341 -> [_ w356]
              frame True {
              }
              frame False {
                n219 = property on="Items" class="Ring (strict)"() -> ("Strings []"=w352:string[])  [unwired: 2 in, 2 out]
                n220 = control-ref of="This VI"() -> (w361:refnum<vi>)
                n221 = call "CRYGlobal Manipulate.vi"("Type"=enum16{"Curves", "Values", "Results", "WFM"}."Curves", "sOption"="byNames", "sAction"="GetGlobal", "sData"=w352) -> ("Curves Out"=w358:T12[])  [unwired: 5 in, 6 out]
                n222 = for {
                  tunnel: w361 -> [w386]
                  tunnel: w358 -> [w364] mode=indexing
                  tunnel: [w363] -> w357 mode=indexing
                  tunnel: w356 -> [w362]
                  i -> [w370]
                  n223 = call "CRYGet Line Infor.vi"("This VI"=w386, "Active Plot Number"=w370, "Graph Type"="POLAR", "XY Graph Control Ref"=w362, "Property Set?"=FALSE) -> ("Line"=w365:u32, "Point/Fill"=w366:u32, "Fill to"=w367:i16, "LineStyle"=w377:string, "LineWidth"=w373:string, "PointStyle"=w372:string, "Interpolation"=w371:string)  [unwired: 16 in]
                  n224 = Match Pattern(string=w377, regular expression="LineStyle") -> (after substring=w383:string)  [unwired: 4 out]
                  n225 = Match Pattern(string=w373, regular expression="LineWidth") -> (after substring=w384:string)  [unwired: 4 out]
                  n226 = Match Pattern(string=w372, regular expression="PointStyle") -> (after substring=w382:string)  [unwired: 4 out]
                  n227 = Match Pattern(string=w371, regular expression="Interpolation") -> (after substring=w379:string)  [unwired: 4 out]
                  n228 = Decimal String To Number(string=w383) -> (number=w376:i32)  [unwired: 3 out]
                  n229 = Decimal String To Number(string=w384) -> (number=w375:i32)  [unwired: 3 out]
                  n230 = Decimal String To Number(string=w382) -> (number=w374:i32)  [unwired: 3 out]
                  n231 = Decimal String To Number(string=w379) -> (number=w369:i32)  [unwired: 3 out]
                  n232 = Bundle By Name(cluster=w364, "Plot Settings.Color"=w365, "Plot Settings.Point Color"=w366, "Plot Settings.Fill To"=w367, "Plot Settings.Line Style"=w376, "Plot Settings.Line Width"=w375, "Plot Settings.Point Style"=w374, "Plot Settings.Interpolation"=w369) -> (w363:T12)
                }
                n233 = call "CRYGlobal Manipulate.vi"("Type"=enum16{"Curves", "Values", "Results", "WFM"}."Curves", "sOption"="byNames", "sAction"="Replace", "sData"=w352, "Curves"=w357) -> ()  [unwired: 4 in, 7 out]
              }
            }
          }
          frame #1 {
            n234 = local read "No Data"() -> (w388:bool)
            n235 = control-ref of="This VI"() -> (w389:refnum<vi>)
            n236 = case shown="False" w388 {
              tunnel: w389 -> [w390 _]
              frame False {
                n237 = local read "Interpolation"() -> (w391:string)
                n238 = local read "LineWidth"() -> (w393:string)
                n239 = local read "PointStyle"() -> (w392:string)
                n240 = local read "LineStyle"() -> (w394:string)
                n241 = To Variant(anything=FALSE) -> (Variant=w396:variant)
                n242 = invoke class="VI" method="Ctrl Val.Set"(reference=w390, "Control Name"=w394, "Value"=w396) -> ()  [unwired: 2 in, 5 out]
                n243 = invoke class="VI" method="Ctrl Val.Set"(reference=w390, "Control Name"=w393, "Value"=w396) -> ()  [unwired: 2 in, 5 out]
                n244 = invoke class="VI" method="Ctrl Val.Set"(reference=w390, "Control Name"=w392, "Value"=w396) -> ()  [unwired: 2 in, 5 out]
                n245 = invoke class="VI" method="Ctrl Val.Set"(reference=w390, "Control Name"=w391, "Value"=w396) -> ()  [unwired: 2 in, 5 out]
              }
              frame True {
              }
            }
          }
        }
        n246 = property class="Bool (strict)"(reference=w338, "Value"=FALSE) -> ()  [unwired: 1 in, 2 out]
        n247 = local read "Discrete/Range"() -> (w340:u16)
        n248 = case shown="1" w340 {
          tunnel: [TRUE ("NewVal") w421] -> w335
          tunnel: [0 w418] -> w336
          frame 0, Default {
          }
          frame 1 {
            n249 = local read "CurValues"() -> (w422:dbl[])
            n250 = local read "CurIndex"() -> (w420:u16)
            n251 = Increment(x=w420) -> (x+1=w419:u16)
            n252 = Index Array(array=w422, index #1=w419, index #2=w420) -> (element #1=w423:dbl, element #2=w424:dbl)
            n253 = Subtract(x=w423, y=w424) -> (x-y=w425:dbl)
            n254 = Greater Or Equal To 0?(x=w425) -> (x >= 0?=w426:bool)
            n255 = case shown="False" w426 {
              tunnel: [FALSE ("NewVal") TRUE ("NewVal")] -> w421
              tunnel: [2 1] -> w418
              frame False {
                n256 = call "CRYGet Error Message.vi"("Error No"=1, "Kind"="Graph") -> ("Message"=w432:string, "Window Title"=w433:string)  [unwired: 4 in, 4 out]
                n257 = call "CRYMessage Dialog.vi"("Window Title"=w433, "YesNoCancel"=T9."OK", "Message Content"=w432) -> ()  [unwired: 7 in, 2 out]
              }
              frame True {
              }
            }
          }
        }
        n258 = flat-sequence {
          tunnel: [w398] -> w337
          tunnel: w336 -> [w398]
          tunnel: w335 -> [w397]
          tunnel: [w397] -> w334
          tunnel: w337 -> [w410]
          tunnel: w334 -> [w409]
          tunnel: [w409] -> w332
          frame #0 {
            n259 = case shown="True" w397 {
              frame False {
              }
              frame True {
                w400 = FALSE ("Caption.Visible")
                n260 = local read "CurValuesRef"() -> (w402:refnum<vi>[])
                n261 = local read "CruColorsRef"() -> (w403:refnum<vi>[])
                n262 = property on="CurValue0_1" class="Bool (strict)"("Visible"=FALSE ("Value (Signaling)")) -> ()  [unwired: 2 in, 2 out]
                n263 = for {
                  tunnel: w403 -> [w408] mode=indexing
                  tunnel: w402 -> [w406] mode=indexing
                  n264 = property class="DigNum (strict)"(reference=w406, "Visible"=FALSE) -> ()  [unwired: 1 in, 2 out]
                  n265 = property class="ColBox"(reference=w408, "Visible"=FALSE) -> ()  [unwired: 1 in, 2 out]
                }
                n266 = property on="CurIndex" class="DigNum (strict)"("Visible"=FALSE) -> ()  [unwired: 2 in, 2 out]
                n267 = property on="CurValue0" class="DigNum (strict)"("Caption.Visible"=w400) -> ()  [unwired: 2 in, 2 out]
                n268 = property on="CurValue1" class="DigNum (strict)"("Caption.Visible"=w400) -> ()  [unwired: 2 in, 2 out]
              }
            }
            n269 = local write "FreqUpdate"(TRUE ("FreqUpdate")) -> ()
            n270 = local write "EndbyOK"(w397) -> ()
          }
          frame #1 {
            n271 = disable-structure shown="Disabled" {
              disable-tunnel: w410 -> [w411 _]
              frame Disabled {
                n272 = case shown="0" w411 {
                  frame 0 {
                    n273 = property on="Draw" class="Bool (strict)"("Val(Sgnl)"=TRUE ("Value (Signaling)")) -> ()  [unwired: 2 in, 2 out]
                  }
                  frame 1 {
                    n274 = property on="Draw" class="Bool (strict)"("Val(Sgnl)"=TRUE ("Value (Signaling)")) -> ()  [unwired: 2 in, 2 out]
                    n275 = property on="CurColValPlot" class="Bool (strict)"("Val(Sgnl)"=TRUE) -> ()  [unwired: 2 in, 2 out]
                  }
                  frame Default {
                    n276 = local write "FreqUpdate"(FALSE ("FreqUpdate")) -> ()
                  }
                }
              }
              frame Enabled {
              }
            }
          }
        }
      }
      event "Polar Tab": Value Change {
        n277 = event-data() -> ("NewVal"=w436:enum32{"Title", "Plot", "XY Graph"})  [unwired: 6 out]
        n278 = case shown="\"Plot\"" w436 {
          frame "Title", Default {
          }
          frame "Plot" {
            n279 = local read "Auto Increment"() -> (w442:bool)
            n280 = local read "Auto/Manual"() -> (w441:u16)
            n281 = Equal To 0?(x=w441) -> (x = 0?=w440:bool)
            n282 = Not(x=w442) -> (.not. x?=w443:bool)
            n283 = property on="Total Rotatin (deg)" class="DigNum (strict)"("Visible"=w442) -> ()  [unwired: 2 in, 2 out]
            n284 = Select(t=T3."Disabled and Grayed Out" ("Disabled"), s=w440, f=T3."Enabled" ("Disabled")) -> (s? t:f=w439:T3)
            n285 = property on="Angle Increment (deg)" class="DigNum (strict)"("Visible"=w443) -> ()  [unwired: 2 in, 2 out]
            n286 = property on="Maximum" class="DigNum (strict)"("DisabledEnum"=w439) -> ()  [unwired: 2 in, 2 out]
            n287 = property on="Minimum" class="DigNum (strict)"("DisabledEnum"=w439) -> ()  [unwired: 2 in, 2 out]
          }
        }
      }
      event "Title Name": Value Change {
        n288 = event-data() -> ("NewVal"=w447:string)  [unwired: 6 out]
        n289 = call "CRYGraph View Socket Client.vi"("sOption"=w447, "nData"=w446, "sData"=w445, "sAction"="SET_GRAPHDATA") -> ()  [unwired: 4 in, 4 out]
      }
      event "Draw": Value Change {
        n290 = event-data() -> ()  [unwired: 7 out]
        n291 = local read "Angle Increment (deg)"() -> (w475:i32)
        n292 = local read "Total Rotatin (deg)"() -> (w470:i32)
        n293 = local read "Background Color"() -> (w448:u32)
        n294 = local read "Zero Adjust (deg)"() -> (w476:i32)
        n295 = local read "Auto Increment"() -> (w473:bool)
        n296 = local read "Discrete/Range"() -> (w468:u16)
        n297 = local read "Visible Section"() -> (w478:u16)
        n298 = local read "Auto/Manual"() -> (w477:u16)
        n299 = local read "Show Name"() -> (w466:bool)
        n300 = local read "PrecisionPolar"() -> (w479:u8)
        n301 = local read "Clip to min"() -> (w482:bool)
        n302 = local read "Line Width"() -> (w451:u16)
        n303 = local read "Grid Color"() -> (w480:u32)
        n304 = local read "CurValues"() -> (w463:dbl[])
        n305 = local read "CurColors"() -> (w469:u32[])
        n306 = local read "Maximum"() -> (w484:dbl)
        n307 = local read "Line Style"() -> (w450:u16)
        n308 = local read "CurIndex"() -> (w467:u16)
        n309 = local read "Minimum"() -> (w483:dbl)
        n310 = local read "Mirror"() -> (w474:bool)
        n311 = local read "Log"() -> (w481:bool)
        n312 = local read "Polar Property"() -> (w485:T1)
        n313 = Bundle By Name(cluster=w485, "polar attributes.maximum"=w484, "polar attributes.minimum"=w483, "polar attributes.clip to min"=w482, "polar attributes.log"=w481, "polar attributes.grid color"=w480, "polar attributes.fmt and prec.format"=T10."Decimal", "polar attributes.fmt and prec.precision"=w479, "polar attributes.visible section"=w478, "Auto/Manual"=w477, "Zero Adjust (deg)"=w476, "Angle Increment (deg)"=w475, "Mirror"=w474, "Auto Increment"=w473, "Total Rotatin (deg)"=w470, "CurValues"=w463, "CurColors"=w469, "Discrete/Rannge"=w468, "CurIndex"=w467, "Show Name"=w466, "Pen.Width"=w451, "Pen.Style"=w450, "BackgroundColor"=w448) -> (w472:T1)
        n314 = Array Size(array=w463) -> (size(s)=w464:i32)
        n315 = invoke class="VI" method="Ctrl Val.Set"(reference=w462, "Control Name"="Polar Property", "Value"=w472) -> (reference out=w449:refnum<vi>)  [unwired: 2 in, 4 out]
        n316 = invoke class="VI" method="Ctrl Val.Set"(reference=w462, "Control Name"="TotalPlotPolar", "Value"=w464) -> ()  [unwired: 2 in, 5 out]
        n317 = local read "XYCursorChange"() -> (w453:string)
        n318 = local read "Dis/RanFreqUpdate"() -> (w452:bool)
        n319 = local read "FreqUpdate"() -> (w458:bool)
        n320 = local read "EndbyOK"() -> (w456:bool)
        n321 = case shown="Default" w453 {
          selector: w453 -> [_ w488]
          tunnel: w449 -> [_ w490]
          frame "" {
          }
          frame Default {
            n322 = local write "XYCursorChange"("" ("XYCursorChange")) -> ()
            n323 = call "CRYGet String Reference.vi"("Label Name"="XYCursor", "VI Refnum"=w490) -> ("String Ref Out"=w489:refnum<vi>)  [unwired: 7 in, 2 out]
            n324 = property class="Str"(reference=w489, "Val(Sgnl)"=w488) -> ()  [unwired: 1 in, 2 out]
          }
        }
        n325 = call "CRYPlot Polar Graph.vi"("pGraph VI In"=w449, "sOption"="Replot") -> ("ItemSyms"=w454:i32[], "Freq Color"=w460:u32[], "Freq Name"=w461:string[])  [unwired: 6 in, 1 out]
        n326 = Compound Arithmetic op=OR(w452, w458) -> (w457:bool)
        n327 = case shown="True" w457 {
          tunnel: w461 -> [_ w497]
          tunnel: w460 -> [_ w496]
          tunnel: [w492 w495] -> w455
          tunnel: w456 -> [w492 w495]
          tunnel: w454 -> [_ w494]
          tunnel: w449 -> [_ w493]
          frame False {
          }
          frame True {
            n328 = flat-sequence {
              tunnel: w497 -> [w501]
              tunnel: w496 -> [w500]
              tunnel: w494 -> [w499]
              tunnel: w493 -> [w498]
              frame #0 {
                n329 = call "CRYData View Legend New Insert.vi"("Item Symbols"=w499, "Color Array"=w500, "ItemName Array"=w501, "sOption"="POLAR_XY", "pGraph VI In"=w498) -> ()  [unwired: 7 out]
              }
              frame #1 {
                n330 = local read "Dis/RanFreqUpdate"() -> (w503:bool)
                n331 = case shown="True" w503 {
                  frame False {
                  }
                  frame True {
                    n332 = local write "Dis/RanFreqUpdate"(FALSE ("Dis/RanFreqUpdate")) -> ()
                    n333 = property on="Discrete/Range" class="Slide (strict)"("DisabledEnum"=T3."Enabled" ("Disabled")) -> ()  [unwired: 2 in, 2 out]
                  }
                }
                n334 = local write "FreqUpdate"(FALSE ("FreqUpdate")) -> ()
              }
            }
          }
        }
      }
      event "Visible Section", "Mirror", "Grid Color", "Zero Adjust (deg)", "Line Width", "Maximum", "Minimum", "Log", "Clip to min", "PrecisionPolar", "Line Style", "Background Color": Value Change {
        n335 = event-data() -> ()  [unwired: 7 out]
        n336 = property on="Draw" class="Bool (strict)"("Val(Sgnl)"=TRUE ("Value (Signaling)")) -> ()  [unwired: 2 in, 2 out]
      }
      event "Auto Increment": Value Change {
        n337 = event-data() -> ("NewVal"=w508:bool)  [unwired: 6 out]
        n338 = flat-sequence {
          tunnel: w508 -> [w509]
          frame #0 {
            n339 = Not(x=w509) -> (.not. x?=w510:bool)
            n340 = property on="Total Rotatin (deg)" class="DigNum (strict)"("Visible"=w509) -> ()  [unwired: 2 in, 2 out]
            n341 = property on="Angle Increment (deg)" class="DigNum (strict)"("Visible"=w510) -> ()  [unwired: 2 in, 2 out]
          }
          frame #1 {
            n342 = property on="Draw" class="Bool (strict)"("Val(Sgnl)"=TRUE ("Value (Signaling)")) -> ()  [unwired: 2 in, 2 out]
          }
        }
      }
      event "Total Rotatin (deg)": Value Change {
        n343 = event-data() -> ("NewVal"=w513:i32)  [unwired: 6 out]
        n344 = flat-sequence {
          tunnel: w513 -> [w517]
          tunnel: w512 -> [w515]
          frame #0 {
            n345 = call "CRYGet Legend Name.vi"("MCListbox Refnum"=w515) -> ("Names Out"=w518:string[])  [unwired: 1 in, 9 out]
            n346 = Array Size(array=w518) -> (size(s)=w519:i32)
            n347 = Decrement(x=w519) -> (x-1=w514:i32)
            n348 = Divide(x=w517, y=w514) -> (x/y=w516:dbl)
            n349 = local write "Angle Increment (deg)"(w516) -> ()
          }
          frame #1 {
            n350 = property on="Draw" class="Bool (strict)"("Val(Sgnl)"=TRUE ("Value (Signaling)")) -> ()  [unwired: 2 in, 2 out]
          }
        }
      }
      event "Angle Increment (deg)": Value Change {
        n351 = event-data() -> ("NewVal"=w522:i32)  [unwired: 6 out]
        n352 = flat-sequence {
          tunnel: w522 -> [w525]
          tunnel: w521 -> [w524]
          frame #0 {
            n353 = call "CRYGet Legend Name.vi"("MCListbox Refnum"=w524) -> ("Names Out"=w527:string[])  [unwired: 1 in, 9 out]
            n354 = Array Size(array=w527) -> (size(s)=w528:i32)
            n355 = Decrement(x=w528) -> (x-1=w523:i32)
            n356 = Multiply(x=w523, y=w525) -> (x*y=w526:i32)
            n357 = local write "Total Rotatin (deg)"(w526) -> ()
          }
          frame #1 {
            n358 = property on="Draw" class="Bool (strict)"("Val(Sgnl)"=TRUE ("Value (Signaling)")) -> ()  [unwired: 2 in, 2 out]
          }
        }
      }
      event "Auto/Manual": Value Change {
        n359 = event-data() -> ("NewVal"=w530:u16)  [unwired: 6 out]
        n360 = flat-sequence {
          tunnel: w530 -> [w535]
          frame #0 {
            n361 = Equal To 0?(x=w535) -> (x = 0?=w534:bool)
            n362 = Select(t=2, s=w534, f=0) -> (s? t:f=w533:i32)
            n363 = property on="Maximum" class="DigNum (strict)"("DisabledEnum"=w533) -> ()  [unwired: 2 in, 2 out]
            n364 = property on="Minimum" class="DigNum (strict)"("DisabledEnum"=w533) -> ()  [unwired: 2 in, 2 out]
          }
          frame #1 {
            n365 = property on="Draw" class="Bool (strict)"("Val(Sgnl)"=TRUE ("Value (Signaling)")) -> ()  [unwired: 2 in, 2 out]
          }
        }
      }
      event "CurIndex": Value Change {
        n366 = event-data() -> ("OldVal"=w538:u16, "NewVal"=w537:u16)  [unwired: 5 out]
        n367 = flat-sequence {
          tunnel: w538 -> [w541]
          tunnel: w537 -> [w540]
          frame #0 {
            n368 = local read "CurColors"() -> (w539:u32[])
            n369 = Array Size(array=w539) -> (size(s)=w542:i32)
            n370 = Increment(x=w540) -> (x+1=w543:u16)
            n371 = Greater?(x=w543, y=w542) -> (0:w544:bool)
            n372 = case shown="True" w544 {
              tunnel: w541 -> [_ w545]
              frame False {
              }
              frame True {
                n373 = local write "CurIndex"(w545) -> ()
              }
            }
          }
          frame #1 {
            n374 = property on="CurColValPlot" class="Bool (strict)"("Val(Sgnl)"=TRUE) -> ()  [unwired: 2 in, 2 out]
            n375 = property on="Draw" class="Bool (strict)"("Val(Sgnl)"=TRUE ("Value (Signaling)")) -> ()  [unwired: 2 in, 2 out]
          }
        }
      }
      event "Add": Value Change {
        n376 = event-data() -> ("CtlRef"=w551:refnum<vi>)  [unwired: 1 out]
        n377 = local read "Discrete/Range"() -> (w552:u16)
        n378 = property class="Bool (strict)"(reference=w551, "Value"=FALSE) -> ()  [unwired: 1 in, 2 out]
        n379 = case shown="0, Default" w552 {
          tunnel: w549 -> [w558 _]
          tunnel: w548 -> [_ _]
          frame 0, Default {
            n380 = flat-sequence {
              tunnel: [w565] -> w553
              frame #0 {
                w565 = "Add" ("Value (Signaling)")
                n381 = local write "XYCursorChange"(w565) -> ()
              }
            }
            n382 = property on="Property Node" class="MCListbox"(reference=w558) -> (reference out=w559:refnum<vi>, "ItemNames"=w557:string[][], "ItemSyms"=w560:i32[])  [unwired: 1 in, 1 out]
            n383 = local read "CurValues"() -> (w564:dbl[])
            n384 = Array Size(array=w564) -> (size(s)=w563:i32)
            n385 = Insert Into Array(array=w557, new element=string[] [] ("new element/subarray")) -> (w556:string[][])  [unwired: 2 in]
            n386 = Insert Into Array(array=w560, new element=38) -> (w561:i32[])  [unwired: 1 in]
            n387 = property on="Property Node" class="MCListbox"(reference=w559, "ItemNames"=w556, "ItemSyms"=w561) -> (reference out=w554:refnum<vi>)  [unwired: 1 in, 1 out]
            n388 = case shown="1, Default" w563 {
              tunnel: w554 -> [_ _]
              tunnel: w553 -> [_ _]
              frame 0 {
                n389 = flat-sequence {
                  frame #0 {
                    w571 = FALSE ("Value (Signaling)")
                    n390 = local read "CurValues"() -> (w566:dbl[])
                    n391 = local write "CurValue0"(0.0 ("CurValue0")) -> ()
                    n392 = local write "FreqUpdate"(TRUE ("FreqUpdate")) -> ()
                    n393 = Not(x=w571) -> (.not. x?=w572:bool)
                    n394 = property on="CurValue0" class="DigNum (strict)"("Visible"=w572) -> ()  [unwired: 2 in, 2 out]
                    n395 = property on="CurValue0_1" class="Bool (strict)"("Visible"=w571) -> ()  [unwired: 2 in, 2 out]
                    n396 = Insert Into Array(array=w566, index=0, new element=0.0 ("new element/subarray")) -> (w567:dbl[])
                    n397 = local write "CurValues"(w567) -> ()
                  }
                  frame #1 {
                    n398 = property on="Draw" class="Bool (strict)"("Val(Sgnl)"=TRUE ("Value (Signaling)")) -> ()  [unwired: 2 in, 2 out]
                  }
                }
              }
              frame 1, Default {
                n399 = flat-sequence {
                  frame #0 {
                    n400 = local read "CurColors"() -> (w586:u32[])
                    n401 = local read "CurValues"() -> (w581:dbl[])
                    n402 = global read "CRYCurve Library Global.vi" "Frequency Color"() -> (w575:u32[])
                    n403 = Array Size(array=w586) -> (size(s)=w582:i32)
                    n404 = Array Size(array=w581) -> (size(s)=w580:i32)
                    n405 = Decrement(x=w580) -> (x-1=w579:i32)
                    n406 = Quotient & Remainder(x=w582, y=7) -> (x-y*floor(x/y)=w584:i32)  [unwired: 1 out]
                    n407 = Index Array(array=w581, index=w579) -> (element=w578:dbl)
                    n408 = Index Array(array=w575, index=w584) -> (element=w583:u32)
                    n409 = Multiply(x=w578, y=2.0) -> (x*y=w577:dbl)
                    n410 = Insert Into Array(array=w586, new element=w583) -> (w587:u32[])  [unwired: 1 in]
                    n411 = Insert Into Array(array=w581, new element=w577) -> (w588:dbl[])  [unwired: 1 in]
                    n412 = local write "CurColors"(w587) -> ()
                    n413 = local write "CurValues"(w588) -> ()
                  }
                  frame #1 {
                    n414 = local read "CurColors"() -> (w590:u32[])
                    n415 = local read "CurIndex"() -> (w596:u16)
                    n416 = Array Size(array=w590) -> (size(s)=w595:i32)
                    n417 = Subtract(x=w595, y=w596) -> (x-y=w593:i32)
                    n418 = local write "FreqUpdate"(TRUE ("FreqUpdate")) -> ()
                    n419 = Greater?(x=w593, y=5) -> (0:w592:bool)
                    n420 = case shown="True" w592 {
                      tunnel: w596 -> [w597 w600]
                      tunnel: [w597 w599] -> w591
                      frame False {
                      }
                      frame True {
                        n421 = Increment(x=w600) -> (x+1=w599:u16)
                        n422 = property on="CurIndex" class="DigNum (strict)"("Visible"=TRUE) -> ()  [unwired: 2 in, 2 out]
                      }
                    }
                    n423 = local write "CurIndex"(w591) -> ()
                  }
                  frame #2 {
                    n424 = property on="Draw" class="Bool (strict)"("Val(Sgnl)"=TRUE ("Value (Signaling)")) -> ()  [unwired: 2 in, 2 out]
                    n425 = property on="CurColValPlot" class="Bool (strict)"("Val(Sgnl)"=TRUE) -> ()  [unwired: 2 in, 2 out]
                  }
                }
              }
            }
          }
          frame 1 {
          }
        }
      }
      event "Delete": Value Change {
        n426 = event-data() -> ("CtlRef"=w604:refnum<vi>)  [unwired: 6 out]
        n427 = local read "Discrete/Range"() -> (w606:u16)
        n428 = property class="Bool (strict)"(reference=w604, "Value"=FALSE) -> ()  [unwired: 1 in, 2 out]
        n429 = case shown="0, Default" w606 {
          tunnel: w603 -> [_ _]
          frame 0, Default {
            n430 = flat-sequence {
              tunnel: [w610] -> w607
              frame #0 {
                w610 = "Delete" ("XYCursorChange")
                n431 = local write "XYCursorChange"(w610) -> ()
              }
            }
            n432 = local read "CurColors"() -> (w608:u32[])
            n433 = Array Size(array=w608) -> (size(s)=w609:i32)
            n434 = case shown="1" w609 {
              selector: w609 -> [_ w616 _]
              tunnel: w607 -> [_ _ _]
              frame 1 {
                n435 = flat-sequence {
                  frame #0 {
                    w613 = TRUE ("Value (Signaling)")
                    n436 = local write "FreqUpdate"(TRUE ("FreqUpdate")) -> ()
                    n437 = Not(x=w613) -> (.not. x?=w614:bool)
                    n438 = local write "CurValues"(dbl[] []) -> ()
                    n439 = property on="CurValue0" class="DigNum (strict)"("Visible"=w614) -> ()  [unwired: 2 in, 2 out]
                    n440 = property on="CurValue0_1" class="Bool (strict)"("Visible"=w613) -> ()  [unwired: 2 in, 2 out]
                  }
                  frame #1 {
                    n441 = property on="Draw" class="Bool (strict)"("Val(Sgnl)"=TRUE ("Value (Signaling)")) -> ()  [unwired: 2 in, 2 out]
                  }
                }
              }
              frame 2.. {
                n442 = flat-sequence {
                  tunnel: w616 -> [w625]
                  frame #0 {
                    n443 = local read "CurIndex"() -> (w618:u16)
                    n444 = Not Equal To 0?(x=w618) -> (x != 0?=w622:bool)
                    n445 = Add(x=w618, y=u16 5) -> (x+y=w626:u16)
                    n446 = Increment(x=w618) -> (x+1=w627:u16)
                    n447 = Equal?(x=w625, y=w626) -> (x = y?=w623:bool)
                    n448 = Equal?(x=w625, y=w627) -> (x = y?=w628:bool)
                    n449 = And(x=w623, y=w622) -> (x .and. y?=w621:bool)
                    n450 = Or(x=w628, y=w621) -> (x .or. y?=w620:bool)
                    n451 = Decrement(x=w618) -> (x-1=w619:u16)
                    n452 = Select(t=w619, s=w620, f=w618) -> (s? t:f=w617:u16)
                    n453 = local write "CurIndex"(w617) -> ()
                  }
                  frame #1 {
                    n454 = local read "CurIndex"() -> (w630:u16)
                    n455 = local read "CurValues"() -> (w631:dbl[])
                    n456 = local read "CurColors"() -> (w634:u32[])
                    n457 = local write "FreqUpdate"(TRUE ("FreqUpdate")) -> ()
                    n458 = Delete From Array(array=w634) -> (array with subset deleted=w633:u32[])  [unwired: 2 in, 1 out]
                    n459 = Delete From Array(array=w631) -> (array with subset deleted=w632:dbl[])  [unwired: 2 in, 1 out]
                    n460 = case shown="1, Default" w630 {
                      frame 0 {
                        n461 = property on="CurIndex" class="DigNum (strict)"("Visible"=FALSE) -> ()  [unwired: 2 in, 2 out]
                      }
                      frame 1, Default {
                      }
                    }
                    n462 = local write "CurColors"(w633) -> ()
                    n463 = local write "CurValues"(w632) -> ()
                  }
                  frame #2 {
                    n464 = property on="CurColValPlot" class="Bool (strict)"("Val(Sgnl)"=TRUE) -> ()  [unwired: 2 in, 2 out]
                    n465 = property on="Draw" class="Bool (strict)"("Val(Sgnl)"=TRUE ("Value (Signaling)")) -> ()  [unwired: 2 in, 2 out]
                  }
                }
              }
              frame Default {
              }
            }
          }
          frame 1 {
          }
        }
      }
      event "Show Name": Value Change {
        n466 = event-data() -> ("NewVal"=w643:bool)  [unwired: 6 out]
        n467 = Select(t="ShowName" ("Value (Signaling)"), s=w643, f="HideName" ("Value (Signaling)")) -> (s? t:f=w639:string)
        n468 = call "CRYGet String Reference.vi"("Label Name"="XYCursor", "VI Refnum"=w638) -> ("String Ref Out"=w640:refnum<vi>)  [unwired: 7 in, 2 out]
        n469 = property class="Str"(reference=w640, "Val(Sgnl)"=w639) -> ()  [unwired: 1 in, 2 out]
      }
      event "CurColValPlot": Value Change {
        n470 = event-data() -> ()  [unwired: 7 out]
        n471 = local read "Discrete/Range"() -> (w645:u16)
        n472 = case shown="0, Default" w645 {
          tunnel: [w656 2 ("y")] -> w650
          tunnel: [w651 w659] -> w646
          frame 0, Default {
            # "Discrete"
            n473 = local read "CurColors"() -> (w652:u32[])
            n474 = local read "CurIndex"() -> (w651:u16)
            n475 = Array Size(array=w652) -> (size(s)=w654:i32)
            n476 = Subtract(x=w654, y=w651) -> (x-y=w655:i32)
            n477 = Greater?(x=w655, y=5) -> (0:w653:bool)
            n478 = Select(t=5 ("y"), s=w653, f=w655) -> (s? t:f=w656:i32)
          }
          frame 1 {
            # "Range"
            n479 = local read "CurIndex"() -> (w659:u16)
          }
        }
        n480 = for {
          N: w650 -> [_]
          tunnel: w646 -> [w681]
          tunnel: [w673] -> w647
          i -> [w673]
          n481 = local read "CurValuesRef"() -> (w675:refnum<vi>[])
          n482 = local read "CruColorsRef"() -> (w676:refnum<vi>[])
          n483 = local read "CurColors"() -> (w683:u32[])
          n484 = local read "CurValues"() -> (w682:dbl[])
          n485 = Add(x=w681, y=w673) -> (x+y=w674:i32)
          n486 = Index Array(array=w675, index=w673) -> (element=w671:refnum<vi>)
          n487 = Index Array(array=w683, index=w674) -> (element=w680:u32)
          n488 = Index Array(array=w682, index=w674) -> (element=w679:dbl)
          n489 = Index Array(array=w676, index=w673) -> (element=w672:refnum<vi>)
          n490 = property class="DigNum (strict)"(reference=w671, "Visible"=TRUE, "Value"=w679) -> ()  [unwired: 1 in, 2 out]
          n491 = property class="ColBox"(reference=w672, "Visible"=TRUE, "Value"=w680) -> ()  [unwired: 1 in, 2 out]
        }
        n492 = Subtract(x=4, y=w647) -> (x-y=w648:i32)
        n493 = for {
          N: w648 -> [_]
          tunnel: w647 -> [w667]
          i -> [w669]
          n494 = local read "CurValuesRef"() -> (w664:refnum<vi>[])
          n495 = local read "CruColorsRef"() -> (w665:refnum<vi>[])
          n496 = Increment(x=w669) -> (x+1=w668:i32)
          n497 = Add(x=w667, y=w668) -> (x+y=w663:i32)
          n498 = Index Array(array=w664, index=w663) -> (element=w661:refnum<vi>)
          n499 = Index Array(array=w665, index=w663) -> (element=w662:refnum<vi>)
          n500 = property class="DigNum (strict)"(reference=w661, "Visible"=FALSE) -> ()  [unwired: 1 in, 2 out]
          n501 = property class="ColBox"(reference=w662, "Visible"=FALSE) -> ()  [unwired: 1 in, 2 out]
        }
      }
      event "CurColor0", "CurColor1", "CurColor2", "CurColor3", "CurColor4": Value Change {
        n502 = event-data() -> ("CtlRef"=w685:refnum<vi>, "NewVal"=w684:u32)  [unwired: 5 out]
        n503 = flat-sequence {
          tunnel: w685 -> [w699]
          tunnel: w684 -> [w690]
          frame #0 {
            n504 = property class="ColBox"(reference=w699) -> ("Label.Text"=w696:string)  [unwired: 1 in, 2 out]
            n505 = Match Pattern(string=w696, regular expression="CurColor") -> (after substring=w697:string)  [unwired: 4 out]
            n506 = local read "CurIndex"() -> (w695:u16)
            n507 = Decimal String To Number(string=w697) -> (number=w694:i32)  [unwired: 3 out]
            n508 = To Unsigned Word Integer(number=w694) -> (unsigned 16bit integer=w693:u16)
            n509 = Add(x=w695, y=w693) -> (x+y=w686:u16)
            n510 = local read "CurColors"() -> (w692:u32[])
            n511 = Number To Decimal String(number=w686) -> (decimal integer string=w688:string)  [unwired: 1 in]
            n512 = Concatenate Strings("CurColor" ("Value (Signaling)"), w688) -> (w689:string)
            n513 = Replace Array Subset(array=w692, new element=w690, index=w686) -> (w691:u32[])
            n514 = local write "XYCursorChange"(w689) -> ()
            n515 = local write "CurColors"(w691) -> ()
          }
          frame #1 {
            n516 = local read "Discrete/Range"() -> (w701:u16)
            n517 = Equal To 0?(x=w701) -> (x = 0?=w700:bool)
            n518 = local write "FreqUpdate"(w700) -> ()
          }
          frame #2 {
            n519 = property on="Draw" class="Bool (strict)"("Val(Sgnl)"=TRUE ("Value (Signaling)")) -> ()  [unwired: 2 in, 2 out]
          }
        }
      }
      event "CurValue0", "CurValue1", "CurValue2", "CurValue3", "CurValue4": Value Change {
        n520 = event-data() -> ("CtlRef"=w703:refnum<vi>, "OldVal"=w704:dbl, "NewVal"=w706:dbl)  [unwired: 4 out]
        n521 = flat-sequence {
          tunnel: w703 -> [w721]
          tunnel: w706 -> [w712]
          tunnel: [w707] -> w705
          tunnel: w705 -> [w722]
          tunnel: w704 -> [w724]
          tunnel: w703 -> [w723]
          frame #0 {
            n522 = property class="DigNum (strict)"(reference=w721) -> ("Label.Text"=w718:string)  [unwired: 1 in, 2 out]
            n523 = Match Pattern(string=w718, regular expression="CurValue") -> (after substring=w719:string)  [unwired: 4 out]
            n524 = local write "FreqUpdate"(TRUE ("FreqUpdate")) -> ()
            n525 = local read "CurIndex"() -> (w717:u16)
            n526 = Decimal String To Number(string=w719) -> (number=w716:i32)  [unwired: 3 out]
            n527 = To Unsigned Word Integer(number=w716) -> (unsigned 16bit integer=w715:u16)
            n528 = local read "CurValues"() -> (w714:dbl[])
            n529 = Add(x=w717, y=w715) -> (x+y=w707:u16)
            n530 = Replace Array Subset(array=w714, new element=w712, index=w707) -> (w713:dbl[])
            n531 = Number To Decimal String(number=w707) -> (decimal integer string=w709:string)  [unwired: 1 in]
            n532 = local write "CurValues"(w713) -> ()
            n533 = Concatenate Strings("CurValue" ("Value (Signaling)"), w709) -> (w710:string)
            n534 = local write "XYCursorChange"(w710) -> ()
          }
          frame #1 {
            n535 = local read "Discrete/Range"() -> (w725:u16)
            n536 = case shown="1" w725 {
              tunnel: w722 -> [_ w731]
              tunnel: w724 -> [_ w730]
              tunnel: w723 -> [_ w729]
              frame 0, Default {
                n537 = property on="Draw" class="Bool (strict)"("Val(Sgnl)"=TRUE ("Value (Signaling)")) -> ()  [unwired: 2 in, 2 out]
              }
              frame 1 {
                n538 = local read "CurValues"() -> (w732:dbl[])
                n539 = local read "CurIndex"() -> (w728:u16)
                n540 = Increment(x=w728) -> (x+1=w727:u16)
                n541 = Index Array(array=w732, index #1=w727, index #2=w728) -> (element #1=w736:dbl, element #2=w735:dbl)
                n542 = Subtract(x=w736, y=w735) -> (x-y=w734:dbl)
                n543 = Greater Or Equal To 0?(x=w734) -> (x >= 0?=w733:bool)
                n544 = case shown="True" w733 {
                  tunnel: w732 -> [w742 _]
                  tunnel: w731 -> [w741 _]
                  tunnel: w730 -> [w739 _]
                  tunnel: w729 -> [w740 _]
                  frame False {
                    n545 = flat-sequence {
                      tunnel: w741 -> [w748]
                      tunnel: w742 -> [w749]
                      tunnel: [w749] -> w738
                      tunnel: [w748] -> w737
                      tunnel: w740 -> [w752]
                      tunnel: w739 -> [w751]
                      tunnel: w738 -> [w753]
                      tunnel: w737 -> [w750]
                      frame #0 {
                        n546 = call "CRYGet Error Message.vi"("Error No"=1, "Kind"="Graph") -> ("Message"=w746:string, "Window Title"=w747:string)  [unwired: 4 in, 4 out]
                        n547 = call "CRYMessage Dialog.vi"("Window Title"=w747, "YesNoCancel"=T9."OK", "Message Content"=w746) -> ()  [unwired: 7 in, 2 out]
                      }
                      frame #1 {
                        n548 = property class="DigNum (strict)"(reference=w752, "Value"=w751) -> ()  [unwired: 1 in, 2 out]
                        n549 = Replace Array Subset(array=w753, new element=w751, index=w750) -> (w754:dbl[])
                        n550 = local write "CurValues"(w754) -> ()
                      }
                    }
                  }
                  frame True {
                    n551 = property on="Draw" class="Bool (strict)"("Val(Sgnl)"=TRUE ("Value (Signaling)")) -> ()  [unwired: 2 in, 2 out]
                  }
                }
              }
            }
          }
        }
      }
      event "Discrete/Range": Value Change {
        n552 = event-data() -> ("NewVal"=w759:u16)  [unwired: 1 out]
        n553 = flat-sequence {
          tunnel: w759 -> [w766]
          tunnel: w756 -> [_]
          tunnel: w759 -> [w802]
          tunnel: w758 -> [w800]
          frame #0 {
            n554 = case shown="1" w766 {
              frame 0, Default {
                # "discrete"
                n555 = local read "CurIndex"() -> (w769:u16)
                n556 = Greater Than 0?(x=w769) -> (x > 0?=w768:bool)
                n557 = property on="CurIndex" class="DigNum (strict)"("Visible"=w768) -> ()  [unwired: 2 in, 2 out]
                n558 = local write "XYCursorChange"("DiscreteFromRange" ("XYCursorChange")) -> ()
              }
              frame 1 {
                # "Range"
                n559 = local read "CurValues"() -> (w775:dbl[])
                n560 = local read "CurIndex"() -> (w771:u16)
                n561 = property on="CurIndex" class="DigNum (strict)"("Visible"=FALSE) -> ()  [unwired: 2 in, 2 out]
                n562 = Array Size(array=w775) -> (size(s)=w773:i32)
                n563 = Subtract(x=w773, y=w771) -> (x-y=w772:i32)
                n564 = case shown="0" w772 {
                  tunnel: w771 -> [_ w794 _]
                  frame 0 {
                    w777 = FALSE ("Value (Signaling)")
                    w779 = 0.0 ("new element/subarray")
                    n565 = global read "CRYCurve Library Global.vi" "Frequency Color"() -> (w776:u32[])
                    n566 = local read "CurValues"() -> (w781:dbl[])
                    n567 = local read "CurColors"() -> (w785:u32[])
                    n568 = Not(x=w777) -> (.not. x?=w778:bool)
                    n569 = property on="CurValue0" class="DigNum (strict)"("Visible"=w778) -> ()  [unwired: 2 in, 2 out]
                    n570 = property on="CurValue0_1" class="Bool (strict)"("Visible"=w777) -> ()  [unwired: 2 in, 2 out]
                    n571 = Index Array(array=w776, index=1) -> (element=w782:u32)
                    n572 = Insert Into Array(array=w781, index=0, new element #1=w779, new element #2=w779) -> (w786:dbl[])
                    n573 = Insert Into Array(array=w785, new element=w782) -> (w784:u32[])  [unwired: 1 in]
                    n574 = local write "CurValues"(w786) -> ()
                    n575 = local write "CurColors"(w784) -> ()
                  }
                  frame 1 {
                    n576 = local read "CurValues"() -> (w798:dbl[])
                    n577 = local read "CurColors"() -> (w792:u32[])
                    n578 = global read "CRYCurve Library Global.vi" "Frequency Color"() -> (w787:u32[])
                    n579 = Index Array(array=w798, index=w794) -> (element=w797:dbl)
                    n580 = Array Size(array=w792) -> (size(s)=w788:i32)
                    n581 = Multiply(x=w797, y=2.0) -> (x*y=w795:dbl)
                    n582 = Quotient & Remainder(x=w788, y=7) -> (x-y*floor(x/y)=w790:i32)  [unwired: 1 out]
                    n583 = Insert Into Array(array=w798, new element=w795) -> (w799:dbl[])  [unwired: 1 in]
                    n584 = Index Array(array=w787, index=w790) -> (element=w789:u32)
                    n585 = local write "CurValues"(w799) -> ()
                    n586 = Insert Into Array(array=w792, new element=w789) -> (w793:u32[])  [unwired: 1 in]
                    n587 = local write "CurColors"(w793) -> ()
                  }
                  frame 2.., Default {
                    # "Nothing..."
                  }
                }
                n588 = local write "XYCursorChange"("Range" ("XYCursorChange")) -> ()
              }
            }
            n589 = local write "Dis/RanFreqUpdate"(TRUE ("Dis/RanFreqUpdate")) -> ()
          }
          frame #1 {
            n590 = case shown="0, Default" w802 {
              tunnel: w800 -> [_ w804]
              frame 0, Default {
                n591 = property on="Draw" class="Bool (strict)"("Val(Sgnl)"=TRUE ("Value (Signaling)")) -> ()  [unwired: 2 in, 2 out]
              }
              frame 1 {
                n592 = local read "CurValues"() -> (w811:dbl[])
                n593 = local read "CurIndex"() -> (w806:u16)
                n594 = Increment(x=w806) -> (x+1=w805:u16)
                n595 = Index Array(array=w811, index #1=w805, index #2=w806) -> (element #1=w810:dbl, element #2=w809:dbl)
                n596 = Subtract(x=w810, y=w809) -> (x-y=w808:dbl)
                n597 = Greater Or Equal To 0?(x=w808) -> (x >= 0?=w807:bool)
                n598 = case shown="True" w807 {
                  tunnel: w804 -> [w812 _]
                  frame False {
                    n599 = flat-sequence {
                      tunnel: w812 -> [w818]
                      frame #0 {
                        n600 = call "CRYGet Error Message.vi"("Error No"=1, "Kind"="Graph") -> ("Message"=w816:string, "Window Title"=w817:string)  [unwired: 4 in, 4 out]
                        n601 = call "CRYMessage Dialog.vi"("Window Title"=w817, "YesNoCancel"=T9."OK", "Message Content"=w816) -> ()  [unwired: 7 in, 2 out]
                      }
                      frame #1 {
                        n602 = call "CRYGet String Reference.vi"("Label Name"="XYCursor", "VI Refnum"=w818) -> ("String Ref Out"=w820:refnum<vi>)  [unwired: 7 in, 2 out]
                        n603 = property class="Str"(reference=w820, "Val(Sgnl)"="Range" ("Value (Signaling)")) -> ()  [unwired: 1 in, 2 out]
                      }
                    }
                  }
                  frame True {
                    n604 = property on="Draw" class="Bool (strict)"("Val(Sgnl)"=TRUE ("Value (Signaling)")) -> ()  [unwired: 2 in, 2 out]
                  }
                }
              }
            }
            n605 = property on="CurColValPlot" class="Bool (strict)"("Val(Sgnl)"=TRUE) -> ()  [unwired: 2 in, 2 out]
          }
        }
        n606 = property on="Discrete/Range" class="Slide (strict)"("DisabledEnum"=T3."Disabled and Grayed Out" ("Disabled")) -> (error out=w756:errorcluster)  [unwired: 2 in, 1 out]
        n607 = Equal To 0?(x=w759) -> (x = 0?=w761:bool)
        n608 = Select(t=T3."Enabled" ("Disabled"), s=w761, f=T3."Disabled and Grayed Out") -> (s? t:f=w762:T3)
        n609 = property on="Add" class="Bool (strict)"("DisabledEnum"=w762) -> ()  [unwired: 2 in, 2 out]
        n610 = property on="Delete" class="Bool (strict)"("DisabledEnum"=w762) -> ()  [unwired: 2 in, 2 out]
        n611 = Not(x=w761) -> (.not. x?=w760:bool)
        n612 = property on="CurValue0" class="DigNum (strict)"("Caption.Visible"=w760) -> ()  [unwired: 2 in, 2 out]
        n613 = property on="CurValue1" class="DigNum (strict)"("Caption.Visible"=w760) -> ()  [unwired: 2 in, 2 out]
      }
      event "PolarXY Tab": Value Change {
        n614 = event-data() -> ("NewVal"=w823:enum32{"Format and Precision", "Plot", "Scale"})  [unwired: 6 out]
        n615 = case shown="\"Format and Precision\", Default" w823 {
          frame "Format and Precision", Default {
            n616 = property on="FormatAxis" class="Ring (strict)"("Val(Sgnl)"=u16 0 ("Value (Signaling)")) -> ()  [unwired: 2 in, 2 out]
          }
          frame "Plot" {
          }
        }
      }
      event "FormatAxis": Value Change {
        n617 = event-data() -> ("NewVal"=w841:u16)  [unwired: 6 out]
        n618 = case shown="2" w841 {
          tunnel: w825 -> [w845 w848 w851]
          tunnel: [w844 w846 w849] -> w842
          frame 0, Default {
            n619 = property class="XYGraph"(reference=w845) -> ("XScale.FormatString"=w844:string)  [unwired: 1 in, 2 out]
          }
          frame 1 {
            n620 = property class="XYGraph"(reference=w848, "ActYScl"=0 ("Active Y Scale")) -> ("YScale.FormatString"=w846:string)  [unwired: 1 in, 2 out]
          }
          frame 2 {
            n621 = property class="XYGraph"(reference=w851, "ActYScl"=1 ("Active Y Scale")) -> ("YScale.FormatString"=w849:string)  [unwired: 1 in, 2 out]
          }
        }
        n622 = call "CRYGet Scale Format Info.vi"("FormatString"=w842) -> ("ScaleFormat"=w843:T13)  [unwired: 10 in]
        n623 = Unbundle By Name(w843) -> ("Notation"=w840:i32, "PrecisionType"=w839:u16, "PrecisionDigits"=w838:u16, "Hide trailing zeros"=w837:bool, "Exponent in multiples of 3"=w836:bool, "Field Width"=w835:u16, "PadType"=w834:u16, "Use minimum field width"=w833:bool, "TimeFormat"=w832:u16, "AMFM"=w831:u16, "HMS"=w830:u16, "Digits"=w829:u16, "DateFormat"=w828:u16, "YMD"=w827:u16, "YearShow"=w826:u16)
        n624 = local write "Use minimum field width"(w833) -> ()
        n625 = local write "Exponent in multiples of 3"(w836) -> ()
        n626 = local write "Hide trailing zeros"(w837) -> ()
        n627 = local write "PrecisionDigits"(w838) -> ()
        n628 = local write "PrecisionType"(w839) -> ()
        n629 = local write "Field Width"(w835) -> ()
        n630 = local write "TimeFormat"(w832) -> ()
        n631 = local write "DateFormat"(w828) -> ()
        n632 = property on="NotationXY" class="LstBox (strict)"("Val(Sgnl)"=w840) -> ()  [unwired: 2 in, 2 out]
        n633 = local write "AMFM"(w831) -> ()
        n634 = local write "PadType"(w834) -> ()
        n635 = local write "HMS"(w830) -> ()
        n636 = local write "YMD"(w827) -> ()
        n637 = local write "YearShow"(w826) -> ()
        n638 = local write "Digits"(w829) -> ()
      }
      event "NotationXY": Value Change {
        n639 = event-data() -> ("NewVal"=w854:i32)  [unwired: 6 out]
        n640 = Not Equal?(x=w854, y=9) -> (x != y?=w853:bool)
        n641 = case shown="9" w854 {
          frame Default {
          }
          frame 0, 3 {
            n642 = property on="Exponent in multiples of 3" class="Bool (strict)"("DisabledEnum"=T3."Enabled" ("Disabled")) -> ()  [unwired: 2 in, 2 out]
          }
          frame 1, 2 {
            n643 = property on="Exponent in multiples of 3" class="Bool (strict)"("DisabledEnum"=T3."Disabled and Grayed Out" ("Disabled")) -> ()  [unwired: 2 in, 2 out]
          }
          frame 9 {
            n644 = property on="TimeFormat" class="Ring (strict)"() -> ("Value"=w862:u16)  [unwired: 2 in, 2 out]
            n645 = property on="DateFormat" class="Ring (strict)"() -> ("Value"=w861:u16)  [unwired: 2 in, 2 out]
            n646 = property on="TimeFormat" class="Ring (strict)"("Val(Sgnl)"=w862) -> ()  [unwired: 2 in, 2 out]
            n647 = property on="DateFormat" class="Ring (strict)"("Val(Sgnl)"=w861) -> ()  [unwired: 2 in, 2 out]
          }
        }
        n648 = property on="Use minimum field width" class="Bool (strict)"() -> ("Value"=w856:bool)  [unwired: 2 in, 2 out]
        n649 = property on="PrecisionDigits" class="DigNum (strict)"("Visible"=w853) -> ()  [unwired: 2 in, 2 out]
        n650 = property on="PrecisionType" class="Ring (strict)"("Visible"=w853) -> ()  [unwired: 2 in, 2 out]
        n651 = property on="Hide trailing zeros" class="Bool (strict)"("Visible"=w853) -> ()  [unwired: 2 in, 2 out]
        n652 = property on="Exponent in multiples of 3" class="Bool (strict)"("Visible"=w853) -> ()  [unwired: 2 in, 2 out]
        n653 = property on="Use minimum field width" class="Bool (strict)"("Visible"=w853) -> ()  [unwired: 2 in, 2 out]
        n654 = property on="Field Width" class="DigNum (strict)"("Visible"=w853) -> ()  [unwired: 2 in, 2 out]
        n655 = property on="PadType" class="Ring (strict)"("Visible"=w853) -> ()  [unwired: 2 in, 2 out]
        n656 = property on="SetFormat" class="Bool (strict)"("Val(Sgnl)"=TRUE ("Value (Signaling)")) -> ()  [unwired: 2 in, 2 out]
        n657 = property on="NotationXY" class="LstBox (strict)"("Disabled Items"=i32[] [5, 6, 7]) -> ()  [unwired: 2 in, 2 out]
        n658 = Not(x=w853) -> (.not. x?=w852:bool)
        n659 = property on="Use minimum field width" class="Bool (strict)"("Val(Sgnl)"=w856) -> ()  [unwired: 2 in, 2 out]
        n660 = property on="TimeFormat" class="Ring (strict)"("Visible"=w852) -> ()  [unwired: 2 in, 2 out]
        n661 = property on="AMFM" class="Slide (strict)"("Visible"=w852) -> ()  [unwired: 2 in, 2 out]
        n662 = property on="HMS" class="Slide (strict)"("Visible"=w852) -> ()  [unwired: 2 in, 2 out]
        n663 = property on="Digits" class="DigNum (strict)"("Visible"=w852) -> ()  [unwired: 2 in, 2 out]
        n664 = property on="DateFormat" class="Ring (strict)"("Visible"=w852) -> ()  [unwired: 2 in, 2 out]
        n665 = property on="YMD" class="Slide (strict)"("Visible"=w852) -> ()  [unwired: 2 in, 2 out]
        n666 = property on="YearShow" class="Slide (strict)"("Visible"=w852) -> ()  [unwired: 2 in, 2 out]
      }
      event "PrecisionType", "PrecisionDigits", "Hide trailing zeros", "Exponent in multiples of 3", "PadType": Value Change {
        n667 = event-data() -> ()  [unwired: 7 out]
        n668 = property on="SetFormat" class="Bool (strict)"("Val(Sgnl)"=TRUE ("Value (Signaling)")) -> ()  [unwired: 2 in, 2 out]
      }
      event "Use minimum field width": Value Change {
        n669 = event-data() -> ("NewVal"=w864:bool)  [unwired: 6 out]
        n670 = property on="Field Width" class="DigNum (strict)"() -> ("Value"=w871:u16)  [unwired: 2 in, 2 out]
        n671 = Equal To 0?(x=w871) -> (x = 0?=w868:bool)
        n672 = Select(t=u16 1 ("Field Width"), s=w868, f=w871) -> (s? t:f=w870:u16)
        n673 = Select(t=T3."Enabled" ("Disabled"), s=w864, f=T3."Disabled and Grayed Out") -> (s? t:f=w872:T3)
        n674 = Select(t=w870, s=w864, f=u16 0 ("Field Width")) -> (s? t:f=w873:u16)
        n675 = property on="Field Width" class="DigNum (strict)"("DisabledEnum"=w872) -> ()  [unwired: 2 in, 2 out]
        n676 = property on="PadType" class="Ring (strict)"("DisabledEnum"=w872) -> ()  [unwired: 2 in, 2 out]
        n677 = property on="Field Width" class="DigNum (strict)"("Value"=w873) -> (error out=w875:errorcluster)  [unwired: 2 in, 1 out]
        n678 = property on="SetFormat" class="Bool (strict)"(error in=w875, "Val(Sgnl)"=TRUE ("Value (Signaling)")) -> ()  [unwired: 1 in, 2 out]
      }
      event "Field Width": Value Change {
        n679 = event-data() -> ("NewVal"=w878:u16)  [unwired: 6 out]
        n680 = property on="SetFormat" class="Bool (strict)"("Val(Sgnl)"=TRUE ("Value (Signaling)")) -> ()  [unwired: 2 in, 2 out]
        n681 = Equal To 0?(x=w878) -> (x = 0?=w881:bool)
        n682 = Select(t=T3."Disabled and Grayed Out" ("Disabled"), s=w881, f=T3."Enabled" ("Disabled")) -> (s? t:f=w877:T3)
        n683 = Select(t=FALSE ("x = 0?"), s=w881, f=TRUE ("x = 0?")) -> (s? t:f=w876:bool)
        n684 = property on="Field Width" class="DigNum (strict)"("DisabledEnum"=w877) -> ()  [unwired: 2 in, 2 out]
        n685 = property on="PadType" class="Ring (strict)"("DisabledEnum"=w877) -> ()  [unwired: 2 in, 2 out]
        n686 = property on="Use minimum field width" class="Bool (strict)"("Visible"=w876) -> ()  [unwired: 2 in, 2 out]
      }
      event "TimeFormat": Value Change {
        n687 = event-data() -> ("NewVal"=w887:u16)  [unwired: 6 out]
        n688 = case shown="0, Default" w887 {
          tunnel: [T3."Enabled" ("Disabled") T3."Disabled and Grayed Out" ("Disabled") T3."Disabled and Grayed Out" ("Disabled")] -> w886
          tunnel: [T3."Enabled" ("Disabled") T3."Enabled" ("Disabled") T3."Disabled and Grayed Out" ("Disabled")] -> w885
          frame 0, Default {
            n689 = property on="HMS" class="Slide (strict)"() -> ("Value"=w889:u16)  [unwired: 2 in, 2 out]
            n690 = property on="HMS" class="Slide (strict)"("Val(Sgnl)"=w889) -> ()  [unwired: 2 in, 2 out]
          }
          frame 1 {
          }
          frame 2 {
          }
        }
        n691 = property on="SetFormat" class="Bool (strict)"("Val(Sgnl)"=TRUE ("Value (Signaling)")) -> ()  [unwired: 2 in, 2 out]
        n692 = property on="AMFM" class="Slide (strict)"("DisabledEnum"=w886) -> ()  [unwired: 2 in, 2 out]
        n693 = property on="HMS" class="Slide (strict)"("DisabledEnum"=w886) -> ()  [unwired: 2 in, 2 out]
        n694 = property on="Digits" class="DigNum (strict)"("DisabledEnum"=w885) -> ()  [unwired: 2 in, 2 out]
      }
      event "AMFM", "Digits", "YMD", "YearShow": Value Change {
        n695 = event-data() -> ()  [unwired: 7 out]
        n696 = property on="SetFormat" class="Bool (strict)"("Val(Sgnl)"=TRUE ("Value (Signaling)")) -> ()  [unwired: 2 in, 2 out]
      }
      event "HMS": Value Change {
        n697 = event-data() -> ("NewVal"=w898:u16)  [unwired: 6 out]
        n698 = property on="SetFormat" class="Bool (strict)"("Val(Sgnl)"=TRUE ("Value (Signaling)")) -> ()  [unwired: 2 in, 2 out]
        n699 = Equal To 0?(x=w898) -> (x = 0?=w901:bool)
        n700 = Select(t=T3."Disabled and Grayed Out" ("Disabled"), s=w901, f=T3."Enabled" ("Disabled")) -> (s? t:f=w897:T3)
        n701 = property on="Digits" class="DigNum (strict)"("DisabledEnum"=w897) -> ()  [unwired: 2 in, 2 out]
      }
      event "DateFormat": Value Change {
        n702 = event-data() -> ("NewVal"=w905:u16)  [unwired: 6 out]
        n703 = case shown="0, Default" w905 {
          tunnel: [T3."Enabled" ("Disabled") T3."Disabled and Grayed Out" ("Disabled")] -> w903
          frame 0, Default {
          }
          frame 1, 2 {
          }
        }
        n704 = property on="SetFormat" class="Bool (strict)"("Val(Sgnl)"=TRUE ("Value (Signaling)")) -> ()  [unwired: 2 in, 2 out]
        n705 = property on="YMD" class="Slide (strict)"("DisabledEnum"=w903) -> ()  [unwired: 2 in, 2 out]
        n706 = property on="YearShow" class="Slide (strict)"("DisabledEnum"=w903) -> ()  [unwired: 2 in, 2 out]
      }
      event "Ignore timestamp information": Value Change {
        n707 = event-data() -> ()  [unwired: 7 out]
        n708 = property on="SetFormat" class="Bool (strict)"("Val(Sgnl)"=TRUE ("Value (Signaling)")) -> ()  [unwired: 2 in, 2 out]
      }
      event "SetFormat": Value Change {
        n709 = event-data() -> ()  [unwired: 7 out]
        n710 = local read "NotationXY"() -> (w910:i32)
        n711 = case shown="9" w910 {
          tunnel: w910 -> [w930 _]
          tunnel: [w929 w969] -> w911
          frame 0..3, 5..7, Default {
            # "%[$][-][+][#][^][0][Width][.Precision || _SignificantDigits][{Unit}][<Embedded information>]Conversion"
            n712 = local read "Exponent in multiples of 3"() -> (w926:bool)
            n713 = local read "Use minimum field width"() -> (w923:bool)
            n714 = local read "Hide trailing zeros"() -> (w927:bool)
            n715 = local read "PrecisionDigits"() -> (w921:u16)
            n716 = local read "PrecisionType"() -> (w922:u16)
            n717 = local read "Field Width"() -> (w924:u16)
            n718 = local read "PadType"() -> (w925:u16)
            n719 = Select(t="#" ("format string"), s=w927, f="" ("format string")) -> (s? t:f=w939:string)
            n720 = Select(t="^" ("format string"), s=w926, f="" ("format string")) -> (s? t:f=w942:string)
            n721 = case shown="True" w923 {
              tunnel: w925 -> [_ w956]
              tunnel: w924 -> [_ w951]
              tunnel: [w948 w955] -> w944
              tunnel: [w948 w949] -> w945
              tunnel: [w948 w954] -> w943
              frame False {
                w948 = ""
              }
              frame True {
                n722 = Not Equal To 0?(x=w951) -> (x != 0?=w952:bool)
                n723 = case shown="2" w956 {
                  tunnel: [w957 "" ("format string") "0" ("format string")] -> w955
                  tunnel: [w957 "-" ("format string") "" ("format string")] -> w954
                  frame 0, Default {
                    w957 = "" ("format string")
                  }
                  frame 1 {
                  }
                  frame 2 {
                  }
                }
                n724 = Number To Decimal String(number=w951) -> (decimal integer string=w950:string)  [unwired: 1 in]
                n725 = Select(t=w950, s=w952, f="") -> (s? t:f=w949:string)
              }
            }
            n726 = Number To Decimal String(number=w921) -> (decimal integer string=w928:string)  [unwired: 1 in]
            n727 = Equal?(x=w922, y=u16 0) -> (x = y?=w936:bool)
            n728 = Index Array(array=string[] ["f", "e", "g", "p", "", "x", "o", "b", "", "T"], index=w930) -> (element=w947:string)
            n729 = Select(t="." ("format string"), s=w936, f="_" ("format string")) -> (s? t:f=w946:string)
            n730 = Concatenate Strings("%" ("string"), w943, w939, w942, w944, w945, w946, w928, w947) -> (w929:string)
          }
          frame 9 {
            n731 = local read "DateFormat"() -> (w964:u16)
            n732 = local read "TimeFormat"() -> (w968:u16)
            n733 = local read "YearShow"() -> (w962:u16)
            n734 = local read "AMFM"() -> (w967:u16)
            n735 = local read "Digits"() -> (w965:u16)
            n736 = local read "HMS"() -> (w966:u16)
            n737 = local read "YMD"() -> (w963:u16)
            n738 = Equal?(x=w964, y=u16 2) -> (x = y?=w984:bool)
            n739 = Equal?(x=w968, y=u16 2) -> (x = y?=w983:bool)
            n740 = case shown="0, Default" w968 {
              tunnel: w967 -> [w1043 _ _]
              tunnel: w966 -> [w1041 _ _]
              tunnel: w965 -> [w1027 w1045 _]
              tunnel: [w1030 w1044 w1047] -> w970
              tunnel: w964 -> [_ _ w1052]
              frame 0, Default {
                # "Custom Format"
                n741 = Equal To 0?(x=w1043) -> (x = 0?=w1034:bool)
                n742 = Not Equal To 0?(x=w1027) -> (x != 0?=w1029:bool)
                n743 = Equal To 0?(x=w1041) -> (x = 0?=w1038:bool)
                n744 = Format Into String(format string=":%%S%%%du", w1027) -> (resulting string=w1026:string)  [unwired: 2 in, 1 out]
                n745 = Select(t="%I:%M" ("format string"), s=w1034, f="%H:%M" ("format string")) -> (s? t:f=w1039:string)
                n746 = Select(t=w1026, s=w1029, f=":%S" ("format string")) -> (s? t:f=w1025:string)
                n747 = Select(t="", s=w1038, f=w1025) -> (s? t:f=w1035:string)
                n748 = Select(t=" %p", s=w1034, f="" ("t")) -> (s? t:f=w1031:string)
                n749 = Concatenate Strings(w1039, w1035, w1031) -> (w1030:string)
              }
              frame 1 {
                # "System Format"
                n750 = Format Into String(format string="%%.%dX", w1045) -> (resulting string=w1044:string)  [unwired: 2 in, 1 out]
              }
              frame 2 {
                # "No Used"
                n751 = Equal?(x=w1052, y=u16 2) -> (x = y?=w1050:bool)
                n752 = Select(t="%.3X" ("format string"), s=w1050, f="") -> (s? t:f=w1047:string)
              }
            }
            n753 = case shown="0, Default" w964 {
              tunnel: w963 -> [w993 _ _]
              tunnel: w962 -> [w992 _ _]
              tunnel: [w990 "%x" ("format string") w1019] -> w971
              tunnel: w968 -> [_ _ w1020]
              frame 0, Default {
                # "Custom Format"
                n754 = case shown="2" w992 {
                  tunnel: ["" ("format string") "%y" ("format string") "%Y" ("format string")] -> w991
                  frame 0, Default {
                  }
                  frame 1 {
                  }
                  frame 2 {
                  }
                }
                n755 = case shown="2" w993 {
                  tunnel: w991 -> [w998 w1005 w1013]
                  tunnel: [w1002 w1009 w1017] -> w990
                  frame 0, Default {
                    n756 = Empty String/Path?(string/path=w998) -> (empty?=w1001:bool)
                    n757 = Concatenate Strings("/" ("string"), w998) -> (w999:string)
                    n758 = Select(t=w998, s=w1001, f=w999) -> (s? t:f=w1000:string)
                    n759 = Concatenate Strings("%m/%d" ("format string"), w1000) -> (w1002:string)
                  }
                  frame 1 {
                    n760 = Empty String/Path?(string/path=w1005) -> (empty?=w1008:bool)
                    n761 = Concatenate Strings("/" ("string"), w1005) -> (w1006:string)
                    n762 = Select(t=w1005, s=w1008, f=w1006) -> (s? t:f=w1007:string)
                    n763 = Concatenate Strings("%d/%m" ("format string"), w1007) -> (w1009:string)
                  }
                  frame 2 {
                    n764 = Empty String/Path?(string/path=w1013) -> (empty?=w1016:bool)
                    n765 = Concatenate Strings(w1013, "/" ("string")) -> (w1015:string)
                    n766 = Select(t=w1013, s=w1016, f=w1015) -> (s? t:f=w1012:string)
                    n767 = Concatenate Strings(w1012, "%m/%d" ("format string")) -> (w1017:string)
                  }
                }
              }
              frame 1 {
                # "System Format"
              }
              frame 2 {
                # "No Used"
                n768 = Equal?(x=w1020, y=u16 2) -> (x = y?=w1022:bool)
                n769 = Select(t="%x" ("format string"), s=w1022, f="") -> (s? t:f=w1019:string)
              }
            }
            n770 = Compound Arithmetic op=AND(w984, w983) -> (w976:bool)
            n771 = Compound Arithmetic op=AND(invert w984, w983) -> (w980:bool)
            n772 = Compound Arithmetic op=AND(w984, invert w983) -> (w981:bool)
            n773 = Compound Arithmetic op=AND(invert w984, invert w983) -> (w985:bool)
            n774 = Compound Arithmetic op=OR(w980, w981) -> (w982:bool)
            n775 = Build Array(w976, w982, w985) -> (w977:bool[])
            n776 = Search 1D Array(1D array=w977, element=TRUE) -> (index of element=w979:i32)  [unwired: 1 in]
            n777 = case shown="2" w979 {
              tunnel: [" " ("format string") "" ("format string") "\n" ("format string")] -> w986
              frame 0, Default {
              }
              frame 1 {
              }
              frame 2 {
              }
            }
            n778 = Concatenate Strings("%<" ("string"), w970, w986, w971, ">T" ("string")) -> (w969:string)
          }
        }
        n779 = local read "FormatAxis"() -> (w912:u16)
        n780 = case shown="0, Default" w912 {
          tunnel: w909 -> [w914 w917 w920]
          tunnel: w911 -> [w913 w915 w918]
          frame 0, Default {
            n781 = property class="XYGraph"(reference=w914, "XScale.FormatString"=w913) -> ()  [unwired: 1 in, 2 out]
          }
          frame 1 {
            n782 = property class="XYGraph"(reference=w917, "ActYScl"=0 ("Active Y Scale"), "YScale.FormatString"=w915) -> ()  [unwired: 1 in, 2 out]
          }
          frame 2 {
            n783 = property class="XYGraph"(reference=w920, "ActYScl"=1 ("Active Y Scale"), "YScale.FormatString"=w918) -> ()  [unwired: 1 in, 2 out]
          }
        }
      }
      event "LineStyle0", "LineStyle1", "LineStyle2", "LineStyle3", "LineStyle4": Value Change {
        n784 = event-data() -> ("CtlRef"=w1053:refnum<vi>)  [unwired: 6 out]
        n785 = flat-sequence {
          tunnel: w1053 -> [w1054]
          frame #0 {
            n786 = local write "Plot PropertyCtrl Ref"(w1054) -> ()
          }
          frame #1 {
            n787 = property on="Plot Property" class="Str"("Val(Sgnl)"="LineStyle" ("Value (Signaling)")) -> ()  [unwired: 2 in, 2 out]
          }
        }
      }
      event "LineWidth0", "LineWidth1", "LineWidth2", "LineWidth3", "LineWidth4", "LineWidth5": Value Change {
        n788 = event-data() -> ("CtlRef"=w1056:refnum<vi>)  [unwired: 6 out]
        n789 = flat-sequence {
          tunnel: w1056 -> [w1057]
          frame #0 {
            n790 = local write "Plot PropertyCtrl Ref"(w1057) -> ()
          }
          frame #1 {
            n791 = property on="Plot Property" class="Str"("Val(Sgnl)"="LineWidth" ("Value (Signaling)")) -> ()  [unwired: 2 in, 2 out]
          }
        }
      }
      event "PointStyle0", "PointStyle1", "PointStyle2", "PointStyle3", "PointStyle4", "PointStyle5", "PointStyle6", "PointStyle7", "PointStyle8", "PointStyle9", "PointStyle10", "PointStyle11", "PointStyle12", "PointStyle13", "PointStyle14", "PointStyle15", "PointStyle16": Value Change {
        n792 = event-data() -> ("CtlRef"=w1059:refnum<vi>)  [unwired: 6 out]
        n793 = flat-sequence {
          tunnel: w1059 -> [w1060]
          frame #0 {
            n794 = local write "Plot PropertyCtrl Ref"(w1060) -> ()
          }
          frame #1 {
            n795 = property on="Plot Property" class="Str"("Val(Sgnl)"="PointStyle" ("Value (Signaling)")) -> ()  [unwired: 2 in, 2 out]
          }
        }
      }
      event "Interpolation0", "Interpolation1", "Interpolation2", "Interpolation3", "Interpolation4", "Interpolation5": Value Change {
        n796 = event-data() -> ("CtlRef"=w1062:refnum<vi>)  [unwired: 6 out]
        n797 = flat-sequence {
          tunnel: w1062 -> [w1063]
          frame #0 {
            n798 = local write "Plot PropertyCtrl Ref"(w1063) -> ()
          }
          frame #1 {
            n799 = property on="Plot Property" class="Str"("Val(Sgnl)"="Interpolation" ("Value (Signaling)")) -> ()  [unwired: 2 in, 2 out]
          }
        }
      }
      event "Plot Property": Value Change {
        n800 = event-data() -> ("NewVal"=w1065:string)  [unwired: 6 out]
        n801 = case shown="\"Interpolation\"" w1065 {
          tunnel: [w1072 w1073 w1074 w1075] -> w1067
          frame "LineStyle", Default {
            n802 = local read "LineStyle"() -> (w1072:string)
          }
          frame "LineWidth" {
            n803 = local read "LineWidth"() -> (w1073:string)
          }
          frame "PointStyle" {
            n804 = local read "PointStyle"() -> (w1074:string)
          }
          frame "Interpolation" {
            n805 = local read "Interpolation"() -> (w1075:string)
          }
        }
        n806 = local read "Plot PropertyCtrl Ref"() -> (w1070:refnum<vi>)
        n807 = local read "Graph VI Ref"() -> (w1068:refnum<vi>)
        n808 = control-ref of="This VI"() -> (w1071:refnum<vi>)
        n809 = property on="Items" class="Ring (strict)"() -> ("Value"=w1069:u16)  [unwired: 2 in, 2 out]
        n810 = call "CRYChange Plot Property.vi"("Items"=w1069, "sOption"=w1065, "Control Ref"=w1070, "pProperty VI"=w1071, "pGraph VI In"=w1068, "ControlName In"=w1067) -> ("ControlName Out"=w1066:string)  [unwired: 5 in]
        n811 = case shown="\"Interpolation\"" w1065 {
          tunnel: w1066 -> [w1076 w1077 w1078 w1079]
          frame "LineStyle", Default {
            n812 = local write "LineStyle"(w1076) -> ()
          }
          frame "LineWidth" {
            n813 = local write "LineWidth"(w1077) -> ()
          }
          frame "PointStyle" {
            n814 = local write "PointStyle"(w1078) -> ()
          }
          frame "Interpolation" {
            n815 = local write "Interpolation"(w1079) -> ()
          }
        }
      }
      event "Items": Value Change {
        n816 = event-data() -> ("NewVal"=w1081:u16)  [unwired: 6 out]
        n817 = flat-sequence {
          tunnel: w1082 -> [w1090]
          tunnel: w1081 -> [w1085]
          tunnel: w1080 -> [w1084]
          tunnel: [w1095] -> w1083
          tunnel: w1083 -> [w1104]
          tunnel: w1081 -> [w1105]
          tunnel: w1082 -> [w1103]
          frame #0 {
            n818 = property class="MCListbox"(reference=w1084) -> ("ItemSyms"=w1089:i32[])  [unwired: 1 in, 2 out]
            n819 = Index Array(array=w1089, index=w1085) -> (element=w1087:i32)
            n820 = Equal?(x=w1087, y=38) -> (x = y?=w1086:bool)
            n821 = property class="XYGraph"(reference=w1090, "Active Plot"=w1085, "Plot.Visible?"=w1086) -> ()  [unwired: 1 in, 2 out]
            n822 = local write "Show Plot"(w1086) -> ()
          }
          frame #1 {
            n823 = control-ref of="This VI"() -> (w1095:refnum<vi>)
            n824 = local read "Interpolation"() -> (w1091:string)
            n825 = local read "LineWidth"() -> (w1093:string)
            n826 = local read "PointStyle"() -> (w1092:string)
            n827 = local read "LineStyle"() -> (w1094:string)
            n828 = To Variant(anything=FALSE) -> (Variant=w1097:variant)
            n829 = invoke class="VI" method="Ctrl Val.Set"(reference=w1095, "Control Name"=w1094, "Value"=w1097) -> ()  [unwired: 2 in, 5 out]
            n830 = invoke class="VI" method="Ctrl Val.Set"(reference=w1095, "Control Name"=w1093, "Value"=w1097) -> ()  [unwired: 2 in, 5 out]
            n831 = invoke class="VI" method="Ctrl Val.Set"(reference=w1095, "Control Name"=w1092, "Value"=w1097) -> ()  [unwired: 2 in, 5 out]
            n832 = invoke class="VI" method="Ctrl Val.Set"(reference=w1095, "Control Name"=w1091, "Value"=w1097) -> ()  [unwired: 2 in, 5 out]
          }
          frame #2 {
            n833 = call "CRYGet Line Infor.vi"("This VI"=w1104, "Active Plot Number"=w1105, "Graph Type"="XY", "XY Graph Control Ref"=w1103, "Property Set?"=TRUE) -> ("Line"=w1098:u32, "Point/Fill"=w1099:u32, "Fill to"=w1100:i16, "LineStyle"=w1109:string, "LineWidth"=w1108:string, "PointStyle"=w1107:string, "Interpolation"=w1106:string)  [unwired: 16 in]
            n834 = local write "Interpolation"(w1106) -> ()
            n835 = local write "LineWidth"(w1108) -> ()
            n836 = local write "Point/Fill"(w1099) -> ()
            n837 = local write "LineStyle"(w1109) -> ()
            n838 = local write "PointStyle"(w1107) -> ()
            n839 = local write "Fill to"(w1100) -> ()
            n840 = local write "Line"(w1098) -> ()
          }
        }
      }
      event "Line": Value Change {
        n841 = event-data() -> ("NewVal"=w1112:u32)  [unwired: 6 out]
        n842 = property class="XYGraph"(reference=w1113, "Plot.Plot Color"=w1112) -> ()  [unwired: 1 in, 2 out]
        n843 = property on="Items" class="Ring (strict)"() -> ("Value"=w1116:u16)  [unwired: 2 in, 2 out]
        n844 = Bundle By Name(cluster=T11 {"Row"=0, "Column"=0} ("Active Cell:Active Cell"), "Row"=w1116, "Column"=1) -> (w1115:T11)
        n845 = case shown="Default" w1110 {
          tunnel: w1111 -> [w1121 _]
          tunnel: w1112 -> [w1120 _]
          tunnel: w1116 -> [w1119 _]
          frame Default {
            n846 = call "CRYSet Plot Settings.vi"("sAction"="Color", "Color"=w1120, "Row"=w1119, "Legend Refnum"=w1121, "Type"=enum16{"Curves", "Values", "Results", "WFM"}."Curves") -> ()  [unwired: 2 in, 5 out]
          }
          frame "ViewReport" {
          }
        }
        n847 = property class="MCListbox"(reference=w1111, "ActiveCell"=w1115, "CellBG"=w1112) -> ()  [unwired: 1 in, 2 out]
      }
      event "Point/Fill": Value Change {
        n848 = event-data() -> ("NewVal"=w1125:u32)  [unwired: 6 out]
        n849 = property class="XYGraph"(reference=w1126, "Plot.Fill/Pt. Color"=w1125) -> ()  [unwired: 1 in, 2 out]
        n850 = property on="Items" class="Ring (strict)"() -> ("Value"=w1127:u16)  [unwired: 2 in, 2 out]
        n851 = case shown="Default" w1124 {
          tunnel: w1123 -> [w1131 _]
          tunnel: w1125 -> [w1130 _]
          tunnel: w1127 -> [w1129 _]
          frame Default {
            n852 = call "CRYSet Plot Settings.vi"("sAction"="PointColor", "Color"=w1130, "Row"=w1129, "Legend Refnum"=w1131, "Type"=enum16{"Curves", "Values", "Results", "WFM"}."Curves") -> ()  [unwired: 2 in, 5 out]
          }
          frame "ViewReport" {
          }
        }
      }
      event "Fill to": Value Change {
        n853 = event-data() -> ("NewVal"=w1136:i16)  [unwired: 6 out]
        n854 = property class="XYGraph"(reference=w1135, "Plot.Fill To"=w1136) -> ()  [unwired: 1 in, 2 out]
        n855 = property on="Items" class="Ring (strict)"() -> ("Value"=w1137:u16)  [unwired: 2 in, 2 out]
        n856 = case shown="Default" w1134 {
          tunnel: w1133 -> [w1141 _]
          tunnel: w1137 -> [w1140 _]
          tunnel: w1136 -> [w1138 _]
          frame Default {
            n857 = call "CRYSet Plot Settings.vi"("Fill To"=w1138, "sAction"="FillTo", "Row"=w1140, "Legend Refnum"=w1141, "Type"=enum16{"Curves", "Values", "Results", "WFM"}."Curves") -> ()  [unwired: 2 in, 5 out]
          }
          frame "ViewReport" {
          }
        }
      }
      event "Show Plot": Value Change {
        w1150 = 38
        n858 = event-data() -> ("NewVal"=w1146:bool)  [unwired: 6 out]
        n859 = local read "Items"() -> (w1145:u16)
        n860 = property class="MCListbox"(reference=w1143) -> (reference out=w1148:refnum<vi>, "ItemSyms"=w1153:i32[])  [unwired: 1 in, 1 out]
        n861 = property class="XYGraph"(reference=w1144, "Active Plot"=w1145, "Plot.Visible?"=w1146) -> ()  [unwired: 1 in, 2 out]
        n862 = Index Array(array=w1153, index=w1145) -> (element=w1147:i32)
        n863 = Equal?(x=w1147, y=w1150) -> (x = y?=w1149:bool)
        n864 = Select(t=37, s=w1149, f=w1150) -> (s? t:f=w1152:i32)
        n865 = Replace Array Subset(array=w1153, new element=w1152, index=w1145) -> (w1154:i32[])
        n866 = property class="MCListbox"(reference=w1148, "ItemSyms"=w1154) -> ()  [unwired: 1 in, 2 out]
      }
      event "Axis": Value Change {
        n867 = event-data() -> ("NewVal"=w1170:u16)  [unwired: 6 out]
        n868 = case shown="1" w1170 {
          tunnel: w1169 -> [w1190 w1204 w1218]
          tunnel: [w1189 w1203 w1217] -> w1167
          tunnel: [w1188 w1202 w1216] -> w1166
          tunnel: [w1187 w1201 w1215] -> w1175
          tunnel: [w1186 w1200 w1214] -> w1173
          tunnel: [w1185 w1199 w1213] -> w1162
          tunnel: [w1184 w1198 w1212] -> w1161
          tunnel: [w1183 w1197 w1211] -> w1160
          tunnel: [w1182 w1196 w1210] -> w1159
          tunnel: [w1181 w1195 w1209] -> w1155
          tunnel: [w1180 w1194 w1208] -> w1156
          tunnel: [w1179 w1193 w1207] -> w1157
          tunnel: [w1178 w1191 w1205] -> w1158
          frame 0, Default {
            n869 = property class="XYGraph"(reference=w1190) -> ("XScale.NameLbl.Visible"=w1189:bool, "XScale.Style"=w1188:u8, "XScale.Mapping Mode"=w1187:u8, "XScale.ScaleFit"=w1186:u8, "XScale.Maximum"=w1185:dbl, "XScale.Minimum"=w1184:dbl, "XScale.TickColor"=w1183:u32, "XScale.MinorTickColor"=w1182:u32, "XScale.Text Color"=w1181:u32, "XScale.MajGrdColor"=w1180:u32, "XScale.MnrGrdColor"=w1179:u32, "XScale.NameLbl.Text"=w1178:string)  [unwired: 1 in, 2 out]
          }
          frame 1 {
            n870 = property class="XYGraph"(reference=w1204, "ActYScl"=0 ("Active X Scale")) -> ("YScale.NameLbl.Visible"=w1203:bool, "YScale.Style"=w1202:u8, "YScale.Mapping Mode"=w1201:u8, "YScale.ScaleFit"=w1200:u8, "YScale.Maximum"=w1199:dbl, "YScale.Minimum"=w1198:dbl, "YScale.TickColor"=w1197:u32, "YScale.MinorTickColor"=w1196:u32, "YScale.Text Color"=w1195:u32, "YScale.MajGrdColor"=w1194:u32, "YScale.MnrGrdColor"=w1193:u32, "YScale.NameLbl.Text"=w1191:string)  [unwired: 1 in, 2 out]
          }
          frame 2 {
            n871 = property class="XYGraph"(reference=w1218, "ActYScl"=1 ("Active X Scale")) -> ("YScale.NameLbl.Visible"=w1217:bool, "YScale.Style"=w1216:u8, "YScale.Mapping Mode"=w1215:u8, "YScale.ScaleFit"=w1214:u8, "YScale.Maximum"=w1213:dbl, "YScale.Minimum"=w1212:dbl, "YScale.TickColor"=w1211:u32, "YScale.MinorTickColor"=w1210:u32, "YScale.Text Color"=w1209:u32, "YScale.MajGrdColor"=w1208:u32, "YScale.MnrGrdColor"=w1207:u32, "YScale.NameLbl.Text"=w1205:string)  [unwired: 1 in, 2 out]
          }
        }
        n872 = Not Equal?(x=w1166, y=u8 5 ("X Scale.Scale Fit")) -> (x != y?=w1165:bool)
        n873 = Equal?(x=w1175, y=u8 1 ("X Scale.Scale Fit")) -> (x = y?=w1164:bool)
        n874 = Equal?(x=w1173, y=u8 2 ("X Scale.Scale Fit")) -> (x = y?=w1163:bool)
        n875 = local write "Show scale label"(w1167) -> ()
        n876 = local write "MaximumXY"(w1162) -> ()
        n877 = local write "MinimumXY"(w1161) -> ()
        n878 = local write "Minor grid"(w1157) -> ()
        n879 = local write "Minor tick"(w1159) -> ()
        n880 = local write "Major grid"(w1156) -> ()
        n881 = local write "Show scale"(w1165) -> ()
        n882 = local write "Major tick"(w1160) -> ()
        n883 = local write "Marker text"(w1155) -> ()
        n884 = local write "Axis Name"(w1158) -> ()
        n885 = local write "Autoscale"(w1163) -> ()
        n886 = local write "Scale Style"(w1166) -> ()
        n887 = local write "LogXY"(w1164) -> ()
        n888 = Select(t=u8 2 ("X Scale.Scale Fit"), s=w1163, f=u8 0 ("X Scale.Scale Fit")) -> (s? t:f=w1168:u8)
        n889 = property on="MaximumXY" class="DigNum (strict)"("DisabledEnum"=w1168) -> ()  [unwired: 2 in, 2 out]
        n890 = property on="MinimumXY" class="DigNum (strict)"("DisabledEnum"=w1168) -> ()  [unwired: 2 in, 2 out]
      }
      event "Axis Name": Value Change {
        n891 = event-data() -> ("NewVal"=w1220:string)  [unwired: 6 out]
        n892 = local write "Axis Name"(w1220) -> ()
        n893 = local read "Axis"() -> (w1221:u16)
        n894 = case shown="2" w1221 {
          tunnel: w1219 -> [w1223 w1226 w1229]
          tunnel: w1220 -> [w1222 w1224 w1227]
          frame 0, Default {
            n895 = property class="XYGraph"(reference=w1223, "XScale.NameLbl.Text"=w1222) -> ()  [unwired: 1 in, 2 out]
          }
          frame 1 {
            n896 = property class="XYGraph"(reference=w1226, "ActYScl"=0 ("Active Y Scale"), "YScale.NameLbl.Text"=w1224) -> ()  [unwired: 1 in, 2 out]
          }
          frame 2 {
            n897 = property class="XYGraph"(reference=w1229, "ActYScl"=1 ("Active Y Scale"), "YScale.NameLbl.Text"=w1227) -> ()  [unwired: 1 in, 2 out]
          }
        }
      }
      event "Show scale label": Value Change {
        n898 = event-data() -> ("NewVal"=w1230:bool)  [unwired: 6 out]
        n899 = local read "Axis"() -> (w1232:u16)
        n900 = case shown="2" w1232 {
          tunnel: w1231 -> [w1234 w1237 w1240]
          tunnel: w1230 -> [w1233 w1235 w1238]
          frame 0, Default {
            n901 = property class="XYGraph"(reference=w1234, "XScale.NameLbl.Visible"=w1233) -> ()  [unwired: 1 in, 2 out]
          }
          frame 1 {
            n902 = property class="XYGraph"(reference=w1237, "ActYScl"=0 ("Active Y Scale"), "YScale.NameLbl.Visible"=w1235) -> ()  [unwired: 1 in, 2 out]
          }
          frame 2 {
            n903 = property class="XYGraph"(reference=w1240, "ActYScl"=1 ("Active Y Scale"), "YScale.NameLbl.Visible"=w1238) -> ()  [unwired: 1 in, 2 out]
          }
        }
      }
      event "Show scale": Value Change {
        n904 = event-data() -> ("NewVal"=w1245:bool)  [unwired: 6 out]
        n905 = local read "Scale Style"() -> (w1244:u8)
        n906 = Equal?(x=u8 5 ("X Scale.Scale Fit"), y=w1244) -> (x = y?=w1248:bool)
        n907 = Select(t=u8 0 ("X Scale.Scale Fit"), s=w1248, f=w1244) -> (s? t:f=w1246:u8)
        n908 = Select(t=w1246, s=w1245, f=u8 5 ("X Scale.Scale Fit")) -> (s? t:f=w1243:u8)
        n909 = local write "Scale Style"(w1243) -> ()
        n910 = local read "Axis"() -> (w1242:u16)
        n911 = case shown="0, Default" w1242 {
          tunnel: w1243 -> [w1252 w1254 w1256]
          tunnel: w1241 -> [w1251 w1255 w1258]
          frame 0, Default {
            n912 = property class="XYGraph"(reference=w1251, "XScale.Style"=w1252) -> ()  [unwired: 1 in, 2 out]
          }
          frame 1 {
            n913 = property class="XYGraph"(reference=w1255, "ActYScl"=0 ("Active Y Scale"), "YScale.Style"=w1254) -> ()  [unwired: 1 in, 2 out]
          }
          frame 2 {
            n914 = property class="XYGraph"(reference=w1258, "ActYScl"=1 ("Active Y Scale"), "YScale.Style"=w1256) -> ()  [unwired: 1 in, 2 out]
          }
        }
      }
      event "LogXY": Value Change {
        n915 = event-data() -> ("NewVal"=w1261:bool)  [unwired: 6 out]
        n916 = Select(t=u8 1 ("X Scale.Scale Fit"), s=w1261, f=u8 0 ("X Scale.Scale Fit")) -> (s? t:f=w1264:u8)
        n917 = local read "Axis"() -> (w1260:u16)
        n918 = case shown="2" w1260 {
          tunnel: w1264 -> [w1266 w1268 w1270]
          tunnel: w1259 -> [w1265 w1269 w1272]
          frame 0, Default {
            n919 = property class="XYGraph"(reference=w1265, "XScale.Mapping Mode"=w1266) -> ()  [unwired: 1 in, 2 out]
          }
          frame 1 {
            n920 = property class="XYGraph"(reference=w1269, "ActYScl"=0 ("Active Y Scale"), "YScale.Mapping Mode"=w1268) -> ()  [unwired: 1 in, 2 out]
          }
          frame 2 {
            n921 = property class="XYGraph"(reference=w1272, "ActYScl"=1 ("Active Y Scale"), "YScale.Mapping Mode"=w1270) -> ()  [unwired: 1 in, 2 out]
          }
        }
      }
      event "GridStyle": Value Change {
        n922 = event-data() -> ("NewVal"=w1275:u16)  [unwired: 6 out]
        n923 = local read "Axis"() -> (w1273:u16)
        n924 = case shown="2" w1273 {
          tunnel: w1275 -> [w1277 w1279 w1281]
          tunnel: w1274 -> [w1276 w1280 w1283]
          frame 0, Default {
            n925 = property class="XYGraph"(reference=w1276, "XScale.Style"=w1277) -> ()  [unwired: 1 in, 2 out]
          }
          frame 1 {
            n926 = property class="XYGraph"(reference=w1280, "ActYScl"=0 ("Active Y Scale"), "YScale.Style"=w1279) -> ()  [unwired: 1 in, 2 out]
          }
          frame 2 {
            n927 = property class="XYGraph"(reference=w1283, "ActYScl"=1 ("Active Y Scale"), "YScale.Style"=w1281) -> ()  [unwired: 1 in, 2 out]
          }
        }
      }
      event "Major tick": Value Change {
        n928 = event-data() -> ("NewVal"=w1285:u32)  [unwired: 6 out]
        n929 = local read "Axis"() -> (w1286:u16)
        n930 = case shown="2" w1286 {
          tunnel: w1284 -> [w1288 w1291 w1294]
          tunnel: w1285 -> [w1287 w1289 w1292]
          frame 0, Default {
            n931 = property class="XYGraph"(reference=w1288, "XScale.TickColor"=w1287) -> ()  [unwired: 1 in, 2 out]
          }
          frame 1 {
            n932 = property class="XYGraph"(reference=w1291, "ActYScl"=0 ("Active Y Scale"), "YScale.TickColor"=w1289) -> ()  [unwired: 1 in, 2 out]
          }
          frame 2 {
            n933 = property class="XYGraph"(reference=w1294, "ActYScl"=1 ("Active Y Scale"), "YScale.TickColor"=w1292) -> ()  [unwired: 1 in, 2 out]
          }
        }
      }
      event "Minor tick": Value Change {
        n934 = event-data() -> ("NewVal"=w1296:u32)  [unwired: 6 out]
        n935 = local read "Axis"() -> (w1297:u16)
        n936 = case shown="0, Default" w1297 {
          tunnel: w1296 -> [w1299 w1301 w1303]
          tunnel: w1295 -> [w1298 w1302 w1305]
          frame 0, Default {
            n937 = property class="XYGraph"(reference=w1298, "XScale.MinorTickColor"=w1299) -> ()  [unwired: 1 in, 2 out]
          }
          frame 1 {
            n938 = property class="XYGraph"(reference=w1302, "ActYScl"=0 ("Active Y Scale"), "YScale.MinorTickColor"=w1301) -> ()  [unwired: 1 in, 2 out]
          }
          frame 2 {
            n939 = property class="XYGraph"(reference=w1305, "ActYScl"=1 ("Active Y Scale"), "YScale.MinorTickColor"=w1303) -> ()  [unwired: 1 in, 2 out]
          }
        }
      }
      event "Marker text": Value Change {
        n940 = event-data() -> ("NewVal"=w1308:u32)  [unwired: 6 out]
        n941 = local read "Axis"() -> (w1307:u16)
        n942 = case shown="0, Default" w1307 {
          tunnel: w1308 -> [w1310 w1312 w1314]
          tunnel: w1306 -> [w1309 w1313 w1316]
          frame 0, Default {
            n943 = property class="XYGraph"(reference=w1309, "XScale.Text Color"=w1310) -> ()  [unwired: 1 in, 2 out]
          }
          frame 1 {
            n944 = property class="XYGraph"(reference=w1313, "ActYScl"=0 ("Active Y Scale"), "YScale.Text Color"=w1312) -> ()  [unwired: 1 in, 2 out]
          }
          frame 2 {
            n945 = property class="XYGraph"(reference=w1316, "ActYScl"=1 ("Active Y Scale"), "YScale.Text Color"=w1314) -> ()  [unwired: 1 in, 2 out]
          }
        }
      }
      event "Major grid": Value Change {
        n946 = event-data() -> ("NewVal"=w1318:u32)  [unwired: 6 out]
        n947 = local read "Axis"() -> (w1319:u16)
        n948 = case shown="0, Default" w1319 {
          tunnel: w1318 -> [w1321 w1323 w1325]
          tunnel: w1317 -> [w1320 w1324 w1327]
          frame 0, Default {
            n949 = property class="XYGraph"(reference=w1320, "XScale.MajGrdColor"=w1321) -> ()  [unwired: 1 in, 2 out]
          }
          frame 1 {
            n950 = property class="XYGraph"(reference=w1324, "ActYScl"=0 ("Active Y Scale"), "YScale.MajGrdColor"=w1323) -> ()  [unwired: 1 in, 2 out]
          }
          frame 2 {
            n951 = property class="XYGraph"(reference=w1327, "ActYScl"=1 ("Active Y Scale"), "YScale.MajGrdColor"=w1325) -> ()  [unwired: 1 in, 2 out]
          }
        }
      }
      event "Minor grid": Value Change {
        n952 = event-data() -> ("NewVal"=w1329:u32)  [unwired: 6 out]
        n953 = local read "Axis"() -> (w1330:u16)
        n954 = case shown="0, Default" w1330 {
          tunnel: w1329 -> [w1332 w1334 w1336]
          tunnel: w1328 -> [w1331 w1335 w1338]
          frame 0, Default {
            n955 = property class="XYGraph"(reference=w1331, "XScale.MnrGrdColor"=w1332) -> ()  [unwired: 1 in, 2 out]
          }
          frame 1 {
            n956 = property class="XYGraph"(reference=w1335, "ActYScl"=0 ("Active Y Scale"), "YScale.MnrGrdColor"=w1334) -> ()  [unwired: 1 in, 2 out]
          }
          frame 2 {
            n957 = property class="XYGraph"(reference=w1338, "ActYScl"=1 ("Active Y Scale"), "YScale.MnrGrdColor"=w1336) -> ()  [unwired: 1 in, 2 out]
          }
        }
      }
      event "Autoscale": Value Change {
        n958 = event-data() -> ("NewVal"=w1344:bool)  [unwired: 6 out]
        n959 = local read "Axis"() -> (w1342:u16)
        n960 = local read "MaximumXY"() -> (w1341:dbl)
        n961 = Select(t=u8 2 ("X Scale.Scale Fit"), s=w1344, f=u8 0 ("X Scale.Scale Fit")) -> (s? t:f=w1347:u8)
        n962 = local read "MinimumXY"() -> (w1340:dbl)
        n963 = Select(t=u8 2 ("X Scale.Scale Fit"), s=w1344, f=u8 0 ("X Scale.Scale Fit")) -> (s? t:f=w1343:u8)
        n964 = case shown="False" w1344 {
          tunnel: w1342 -> [w1353 _]
          tunnel: w1341 -> [w1352 _]
          tunnel: w1340 -> [w1351 _]
          tunnel: w1339 -> [w1350 _]
          frame False {
            n965 = case shown="0, Default" w1353 {
              tunnel: w1350 -> [w1356 w1360 w1364]
              tunnel: w1352 -> [w1355 w1358 w1362]
              tunnel: w1351 -> [w1354 w1357 w1361]
              frame 0, Default {
                n966 = property class="XYGraph"(reference=w1356, "XScale.Maximum"=w1355, "XScale.Minimum"=w1354) -> ()  [unwired: 1 in, 2 out]
              }
              frame 1 {
                n967 = property class="XYGraph"(reference=w1360, "ActYScl"=0 ("Active Y Scale"), "YScale.Maximum"=w1358, "YScale.Minimum"=w1357) -> ()  [unwired: 1 in, 2 out]
              }
              frame 2 {
                n968 = property class="XYGraph"(reference=w1364, "ActYScl"=1 ("Active Y Scale"), "YScale.Maximum"=w1362, "YScale.Minimum"=w1361) -> ()  [unwired: 1 in, 2 out]
              }
            }
          }
          frame True {
          }
        }
        n969 = case shown="2" w1342 {
          tunnel: w1347 -> [w1365 w1368 w1370]
          tunnel: w1339 -> [w1366 w1369 w1372]
          frame 0, Default {
            n970 = property class="XYGraph"(reference=w1366, "XScale.ScaleFit"=w1365) -> ()  [unwired: 1 in, 2 out]
          }
          frame 1 {
            n971 = property class="XYGraph"(reference=w1369, "ActYScl"=0 ("Active Y Scale"), "YScale.ScaleFit"=w1368) -> ()  [unwired: 1 in, 2 out]
          }
          frame 2 {
            n972 = property class="XYGraph"(reference=w1372, "ActYScl"=1 ("Active Y Scale"), "YScale.ScaleFit"=w1370) -> ()  [unwired: 1 in, 2 out]
          }
        }
        n973 = property on="MaximumXY" class="DigNum (strict)"("DisabledEnum"=w1343) -> ()  [unwired: 2 in, 2 out]
        n974 = property on="MinimumXY" class="DigNum (strict)"("DisabledEnum"=w1343) -> ()  [unwired: 2 in, 2 out]
      }
      event "MaximumXY": Value Change {
        n975 = event-data() -> ("NewVal"=w1373:dbl)  [unwired: 6 out]
        n976 = local read "Axis"() -> (w1375:u16)
        n977 = local write "MaximumXY"(w1373) -> ()
        n978 = case shown="0, Default" w1375 {
          tunnel: w1373 -> [w1377 w1379 w1381]
          tunnel: w1374 -> [w1376 w1380 w1383]
          frame 0, Default {
            n979 = property class="XYGraph"(reference=w1376, "XScale.Maximum"=w1377) -> ()  [unwired: 1 in, 2 out]
          }
          frame 1 {
            n980 = property class="XYGraph"(reference=w1380, "ActYScl"=0 ("Active Y Scale"), "YScale.Maximum"=w1379) -> ()  [unwired: 1 in, 2 out]
          }
          frame 2 {
            n981 = property class="XYGraph"(reference=w1383, "ActYScl"=1 ("Active Y Scale"), "YScale.Maximum"=w1381) -> ()  [unwired: 1 in, 2 out]
          }
        }
      }
      event "MinimumXY": Value Change {
        n982 = event-data() -> ("NewVal"=w1384:dbl)  [unwired: 6 out]
        n983 = local read "Axis"() -> (w1386:u16)
        n984 = case shown="0, Default" w1386 {
          tunnel: w1384 -> [w1388 w1390 w1392]
          tunnel: w1385 -> [w1387 w1391 w1394]
          frame 0, Default {
            n985 = property class="XYGraph"(reference=w1387, "XScale.Minimum"=w1388) -> ()  [unwired: 1 in, 2 out]
          }
          frame 1 {
            n986 = property class="XYGraph"(reference=w1391, "ActYScl"=0 ("Active Y Scale"), "YScale.Minimum"=w1390) -> ()  [unwired: 1 in, 2 out]
          }
          frame 2 {
            n987 = property class="XYGraph"(reference=w1394, "ActYScl"=1 ("Active Y Scale"), "YScale.Minimum"=w1392) -> ()  [unwired: 1 in, 2 out]
          }
        }
        n988 = local write "MinimumXY"(w1384) -> ()
      }
    }
  }
  n989 = flat-sequence {
    tunnel: w15 -> [_]
    tunnel: "Graph VI Ref" -> [w1395]
    frame #0 {
      n990 = invoke class="VI" method="Ctrl Val.Set"(reference=w1395, "Control Name"="PropertyLoading", "Value"=FALSE ("FreqUpdate")) -> ()  [unwired: 2 in, 5 out]
    }
  }
